vi "运维调试_氨氮.vi"() -> ()   [LabVIEW 2016, in "斯坦道氨氮.lvlib"]
uses:
  <vilib>/Utility/miscctls.llb/LVPointTypeDef.ctl
  <vilib>/Utility/config.llb/NI_LVConfig.lvlib
  <vilib>/ptbypt/NI_PtbyPt.lvlib
panel:
  in  "定时设置":cluster{"启动":bool, "控制命令":T1, "测量参数":T2}(xcontrol)
  in  "仪器参数设置":bool
  in  "模块启用":bool
  in  "串口设置":bool
  in  "备用系数一键写入":bool
  in  "公式一键写入":bool
  in  "流程路径":path=path "C:/Users/STD/Documents/斯坦道流程文件/流程.xml"
  in  "曲线模型":cluster{"X^2":dbl, "X":dbl, "B":dbl, "r^2":dbl}(xcontrol)
  out "字符串":string
  in  "质控参数设置":bool
  in  "自动测试量程配置":T3
  out "温度2":sgl
  out "温度1":sgl
  out "ADC":sgl
  out "固件版本号":string
  in  "数组":string[](array[string])
  in  "备用系数写入":bool
  in  "备用系数读取":bool
  in  "备用系数":T4
  in  "量程切换阈值写入":bool
  in  "量程切换阈值读取":bool
  in  "量程切换阈值":cluster{"阈值":dbl, "标液浓度":dbl}
  in  "参数下拉列表":enum16{"总磷", "总氮", "氨氮"}(ring)=enum."氨氮"
  in  "量程下拉列表":enum16{"低量程", "高量程"}(ring)
  in  "测量模式下拉列表":enum16{"水样测量", "零点核查", "跨度核查", "标样核查", "加标回收"}(ring)
  in  "公式":cluster{"X^2":dbl, "X":dbl, "b":dbl}
  in  "写公式":bool
  in  "读公式":bool
  in  "返回":bool
  in  "设置":bool
  out "序列号":string="序列号"
  out "测量数据":T5(xcontrol)
  out "集成报警信息":string
  out "运行状态":T6(xcontrol)
  in  "停止":bool
  in  "手动启动":bool
  in  "单步测试":bool
  in  "总磷氨氮调试":u16[](xcontrol)
  out "F3":sgl format="%#.6f"
  out "F2":sgl format="%#.6f"
  out "F1":sgl format="%#.6f"
  out "F0":sgl format="%#.6f"
  out "多列列表框":i32(listbox)
  # "参数设置"
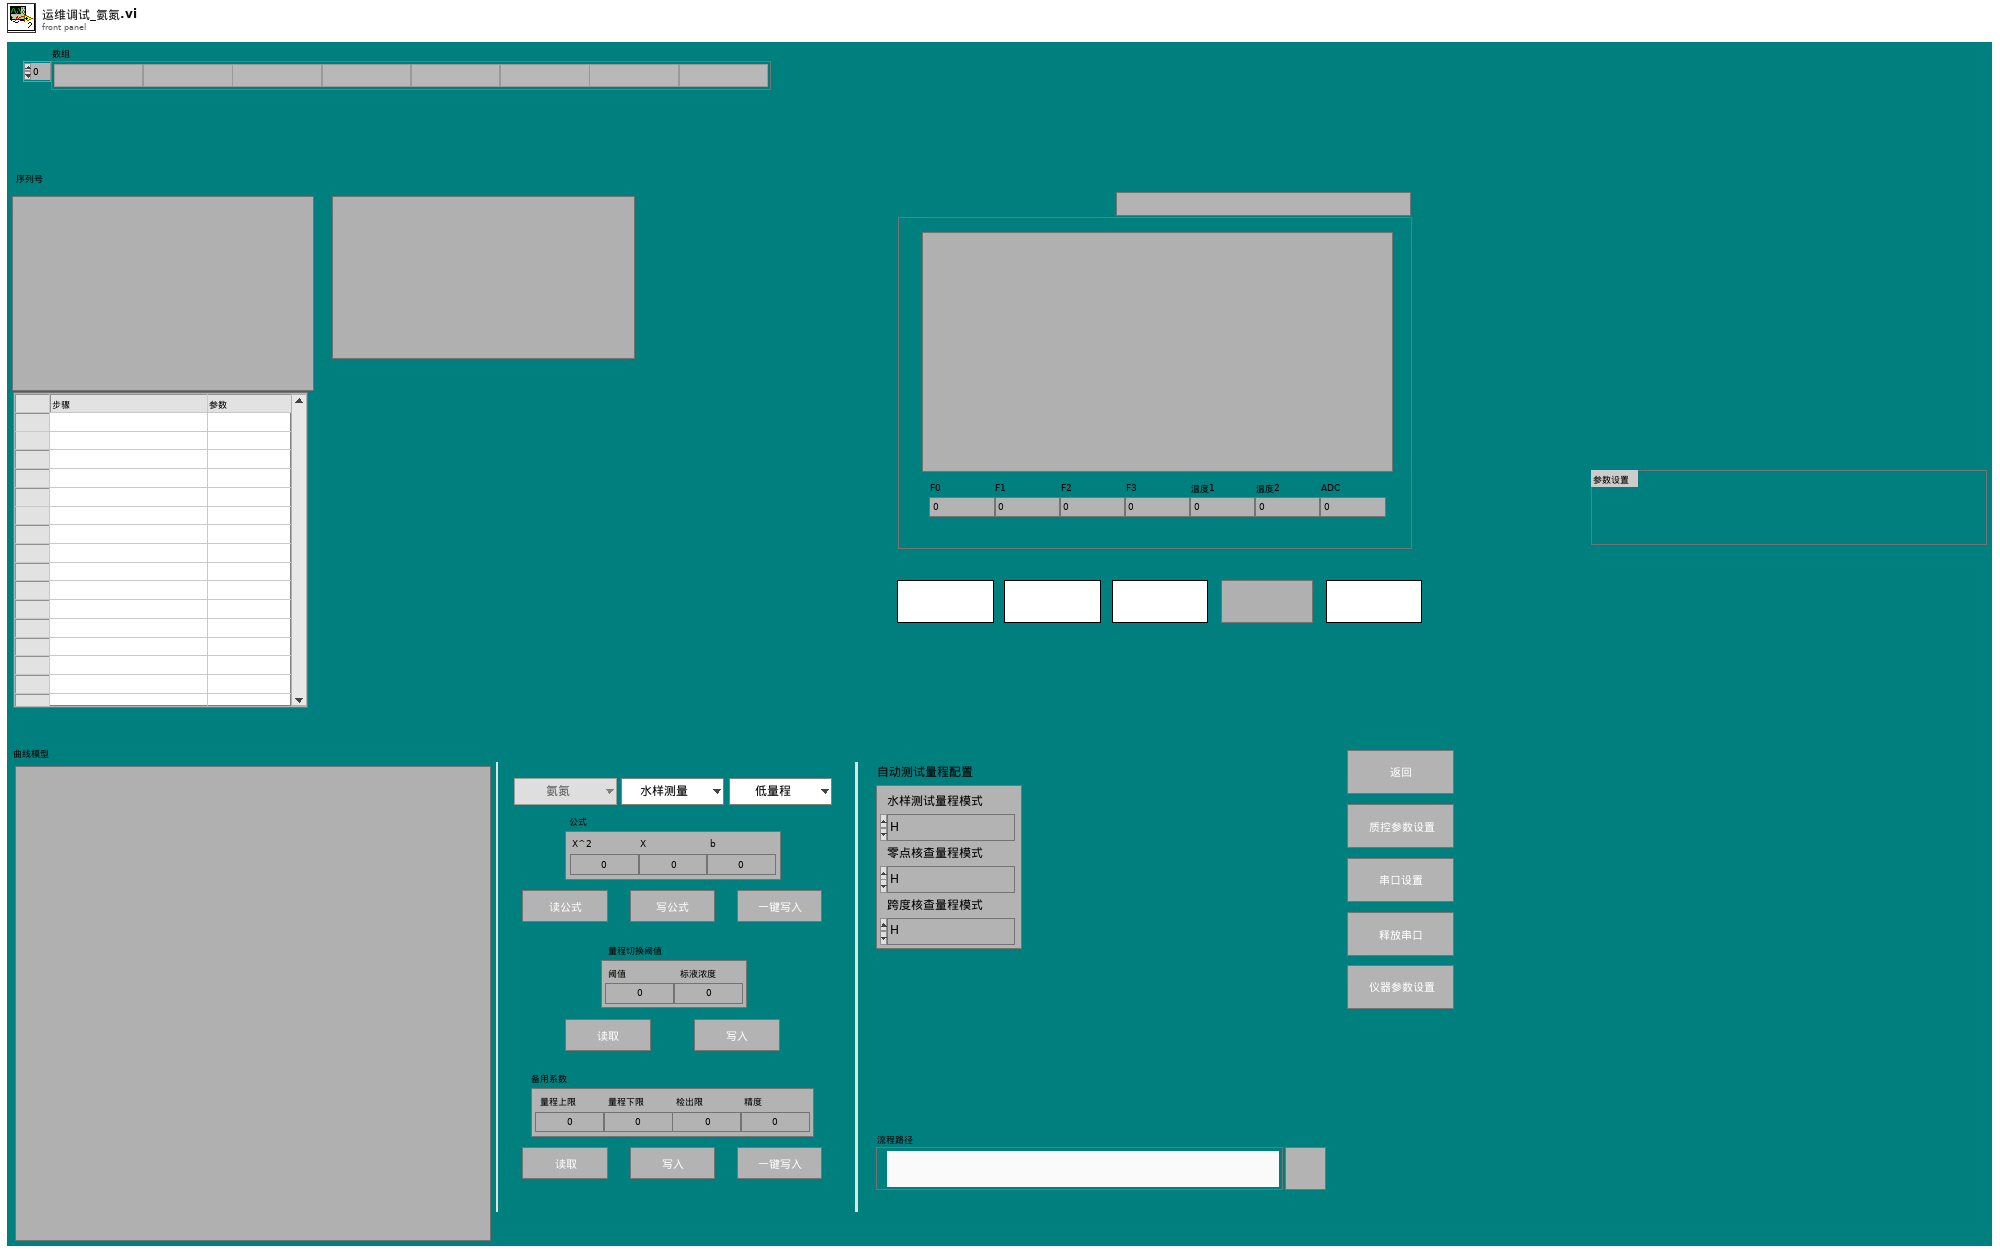
[diagram p1: front panel]
types:
  T1 = typedef "定时设置.xctl/国标控制命令.ctl" = enum16{"启动测量", "标样核查", "零点核查", "跨度核查", "空白测试", "平行样测试", "加标回收", "空白校准", "标样校准", "初始化（清洗）", "停止测试", "仪器重启", "校时", "模式设置", "测量间隔设置"}
  T2 = typedef "定时设置.xctl/测量参数.ctl" = u16
  T3 = cluster{"水样测试量程模式":enum16{"H", "L", "AUTO"}, "空白核查量程模式":enum16{"H", "L", "AUTO"}, "跨度核查量程模式":enum16{"H", "L", "AUTO"}}
  T4 = cluster{"量程上限":dbl, "量程下限":dbl, "检出限":dbl, "精度":dbl}
  T5 = cluster{"flowid":u16, "测量精度":u16, "测量数据区":cluster{"因子编码":u32, "单位":u16, "标样参考值":sgl, "水样数据时间":timestamp, "水样实测值":sgl, "水样数据标识":string, "标样数据时间":timestamp, "标样实测值":sgl, "标样数据标识":string, "空白数据时间":timestamp, "空白实测值":sgl, "空白数据标识":string, "零点核查数据时间":timestamp, "零点核查实测值":sgl, "零点核查数据标识":string, "跨度核查数据时间":timestamp, "跨度核查实测值":sgl, "跨度核查数据标识":string, "加标回收数据时间":timestamp, "加标回收实测值":sgl, "加标回收数据标识":string, "平行样数据时间":timestamp, "平行样实测值":sgl, "平行样数据标识":string, "F0":sgl, "F1":sgl, "F2":sgl, "F3":sgl, "F4":sgl, "F5":sgl, "F6":sgl, "F7":sgl, "温度":sgl, "湿度":sgl, "X值":sgl}}
  T6 = cluster{"系统时间":timestamp, "工作状态":enum16{"空闲", "水样测试", "标样核查", "零点核查", "跨度核查", "空白测试", "平行样测试", "加标回收", "空白校准", "标样校准", "初始化（清洗）"}, "测量模式":enum16{"待机", "连续模式", "周期模式", "定点模式", "受控模式", "手动模式"}, "告警代码":u16, "故障代码":u16, "日志代码":u16, "软件版本":u16, "F0":sgl, "F1":sgl, "F2":sgl, "F3":sgl, "T":sgl, "H":sgl, "id":u16, "flowid":u16, "量程":u16, "总磷控温温度1":sgl, "营养盐控温温度2":sgl, "ADC":sgl}
  T7 = cluster{"时间源选择":enum16{"系统时间源", "仪器时间源"}, "外部时间源":timestamp}
  T8 = enum16{"空闲", "水样测试", "标样核查", "零点核查", "跨度核查", "空白测试", "平行样测试", "加标回收", "空白校准", "标样校准", "初始化（清洗）"}
  T9 = enum32{"Bad", "Idle", "Run top level", "Running"}
  T10 = typedef "LVPointTypeDef.ctl" = cluster{"Horizontal":i16, "Vertical":i16}
  T11 = cluster{"因子编码":u32, "单位":u16, "标样参考值":sgl, "水样数据时间":timestamp, "水样实测值":sgl, "水样数据标识":string, "标样数据时间":timestamp, "标样实测值":sgl, "标样数据标识":string, "空白数据时间":timestamp, "空白实测值":sgl, "空白数据标识":string, "零点核查数据时间":timestamp, "零点核查实测值":sgl, "零点核查数据标识":string, "跨度核查数据时间":timestamp, "跨度核查实测值":sgl, "跨度核查数据标识":string, "加标回收数据时间":timestamp, "加标回收实测值":sgl, "加标回收数据标识":string, "平行样数据时间":timestamp, "平行样实测值":sgl, "平行样数据标识":string, "F0":sgl, "F1":sgl, "F2":sgl, "F3":sgl, "F4":sgl, "F5":sgl, "F6":sgl, "F7":sgl, "温度":sgl, "湿度":sgl, "X值":sgl}
  T12 = typedef "NI_LVConfig.lvlib/Config Data RefNum.ctl" = refnum<k1>
  T13 = cluster{"参数下拉列表":enum16{"总磷", "总氮", "氨氮"}, "测量模式下拉列表":enum16{"水样测量", "零点核查", "跨度核查", "标样核查", "加标回收"}, "量程下拉列表":enum16{"低量程", "高量程"}}
  T14 = cluster{"启动模式":enum16{"跨度核查", "水样测量", "空白核查", "标样核查", "加标回收"}, "启动参数":u16, "量程":enum16{"低量程", "高量程"}}
  T15 = cluster{"时间标识":timestamp, "设备":string, "日志信息":string, "流程参数":string}
  T16 = cluster{"时间标识":timestamp, "设备":string, "日志信息":string}
  T17 = typedef "LVRowAndColumnUnsignedTypeDef.ctl" = cluster{"Row":u32, "Column":u32}
  T18 = cluster{"站号":u16, "量程切换":enum32{"H", "L", "AUTO"}, "控制命令":enum16{"启动测量", "标样核查", "零点核查", "跨度核查", "空白测试", "平行样测试", "加标回收", "空白校准", "标样校准", "初始化（清洗）", "停止测试", "仪器重启", "校时", "模式设置", "测量间隔设置"}, "模式设置":enum16{"待机", "连续模式", "周期模式", "定点模式", "受控模式", "手动模式"}, "测量间隔":u16}
  T19 = cluster{"氨氮跨度值":dbl, "氨氮零点标准液浓度":dbl, "氨氮跨度标准液浓度":dbl, "氨氮标准液标准浓度":dbl}
  T20 = cluster{"确定":bool, "跨度值":dbl, "零点标准液浓度":dbl, "跨度标准液浓度":dbl, "标准液标准浓度":dbl}
  T21 = cluster{"测量量程":dbl, "测量精度":dbl, "测量间隔":dbl, "消解温度":dbl, "消解时长":dbl, "空白校准时间":timestamp, "曲线截距":dbl, "曲线斜率":dbl, "测量检出限":dbl, "测量信号值":dbl, "线性相关系数":dbl, "二次多项式系数":dbl, "标样校准时间":timestamp, "稀释倍数":dbl, "三项式系数":dbl, "空白标定系数":dbl, "量程系数":dbl, "F0/ORPA":dbl, "F1/ORPB":dbl, "F2/ORPK":dbl, "F3":dbl, "F4":dbl, "F5":dbl, "F6":dbl, "F7":dbl, "X0/滴定数":dbl, "量程":dbl}
  T22 = cluster{"确定":bool, "测量量程":dbl, "测量精度":dbl, "测量间隔":dbl, "消解温度":dbl, "消解时长":dbl, "空白校准时间":timestamp, "曲线截距":dbl, "曲线斜率":dbl, "测量检出限":dbl, "测量信号值":dbl, "线性相关系数":dbl, "二次多项式系数":dbl, "标样校准时间":timestamp, "稀释倍数":dbl, "三项式系数":dbl, "空白标定系数":dbl, "量程系数":dbl, "F0/ORPA":dbl, "F1/ORPB":dbl, "F2/ORPK":dbl, "F3":dbl, "F4":dbl, "F5":dbl, "F6":dbl, "F7":dbl, "X0/滴定数":dbl, "量程":dbl}
  T23 = enum8{"Enabled", "Disabled", "Disabled and Grayed Out"}
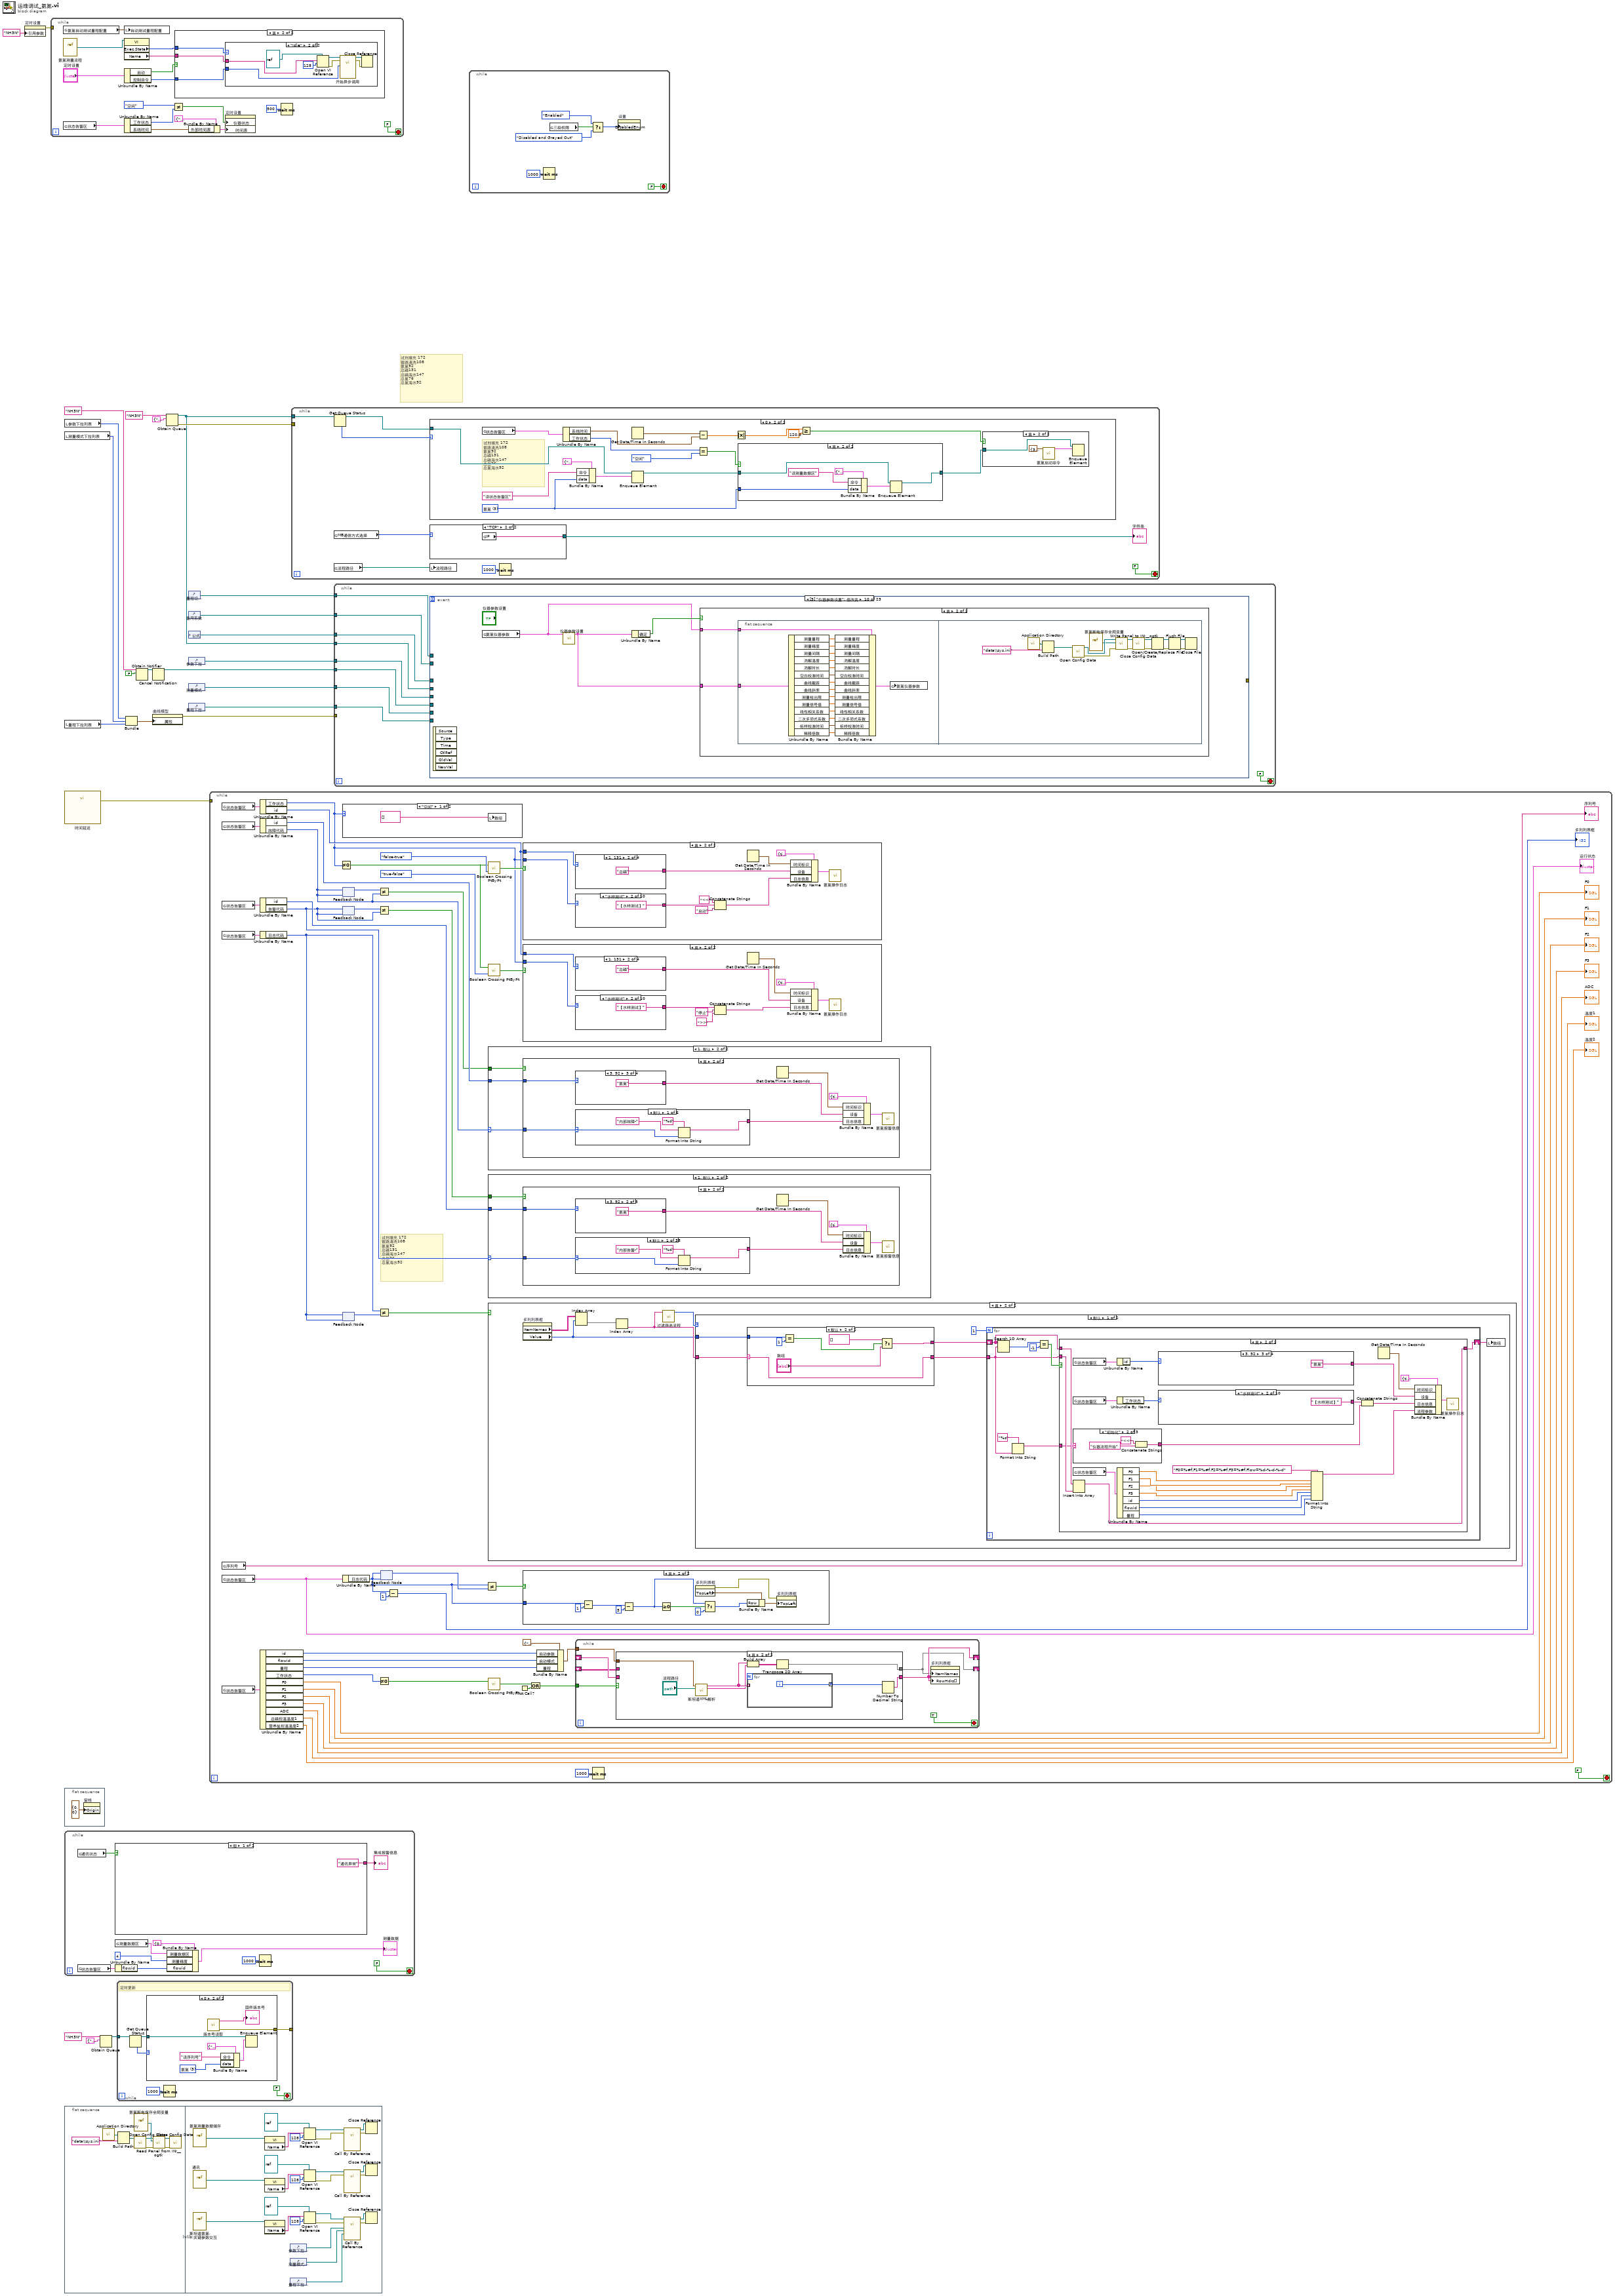
[diagram p0: block diagram]
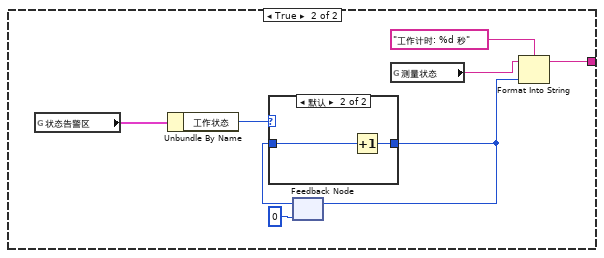
[diagram p3: hidden frame]
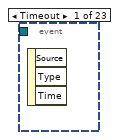
[diagram p7: hidden frame]
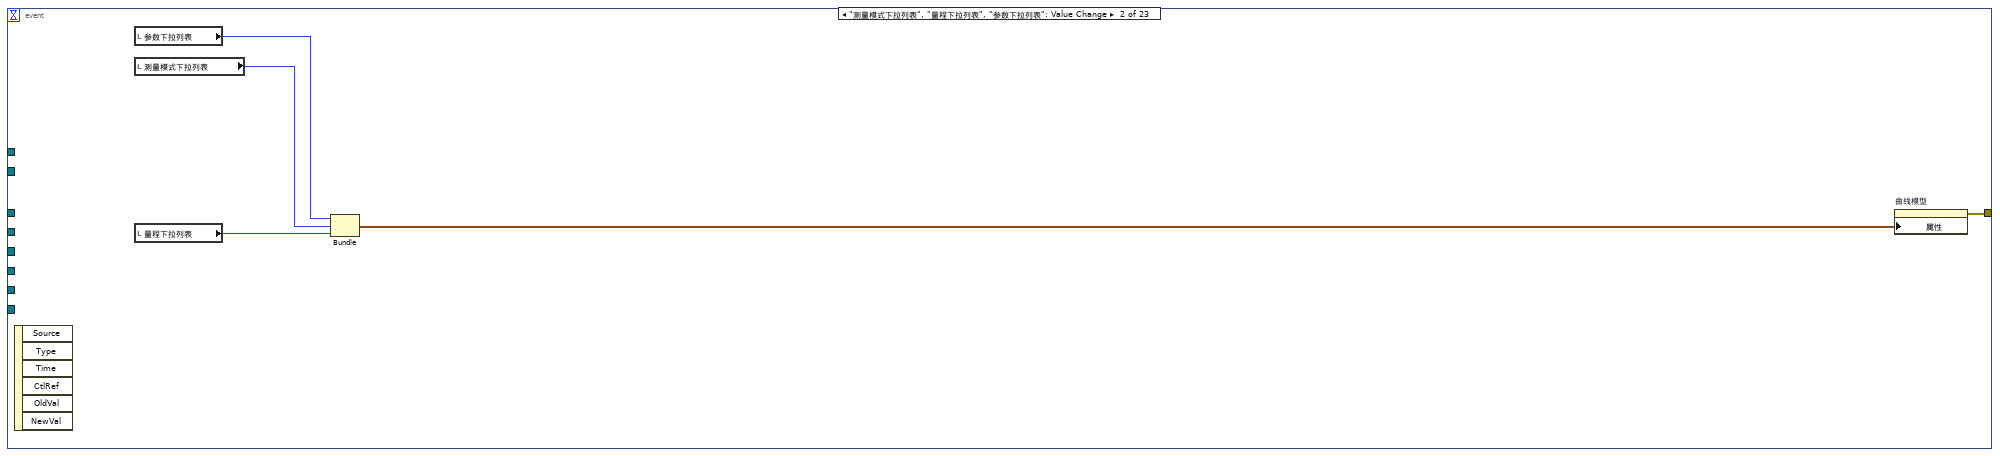
[diagram p8: hidden frame]
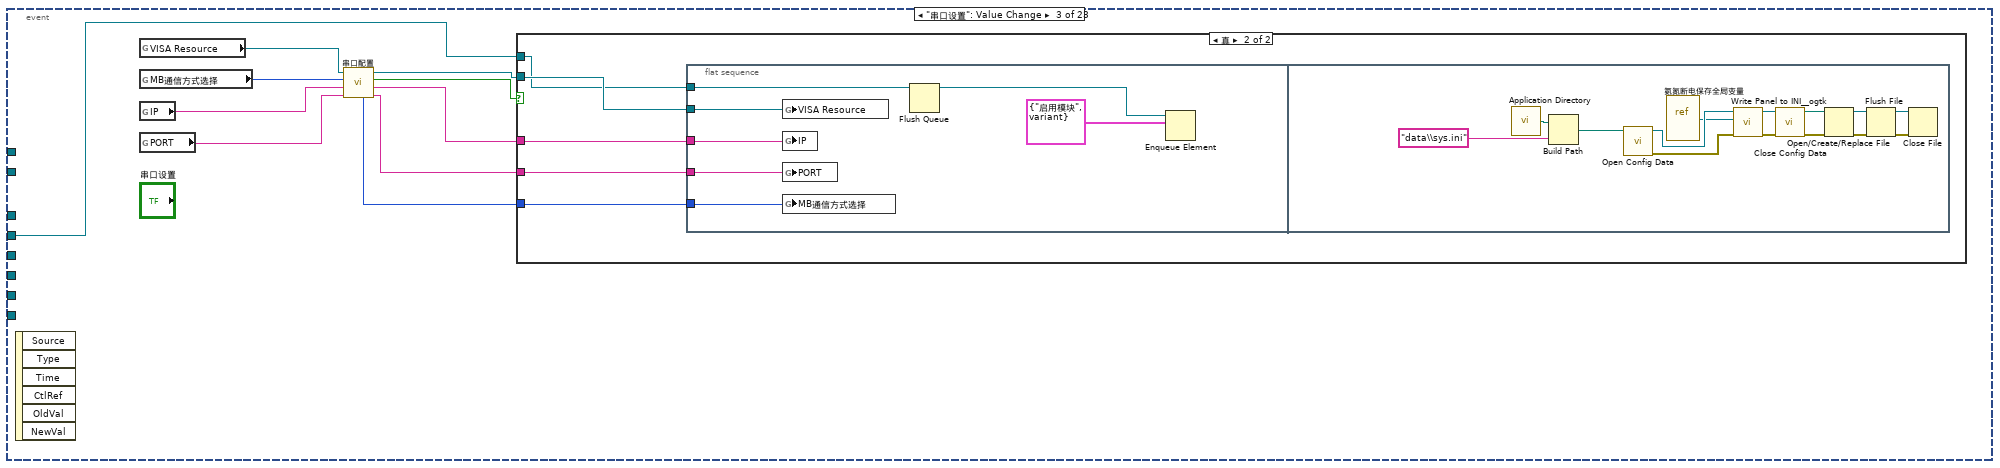
[diagram p9: hidden frame]
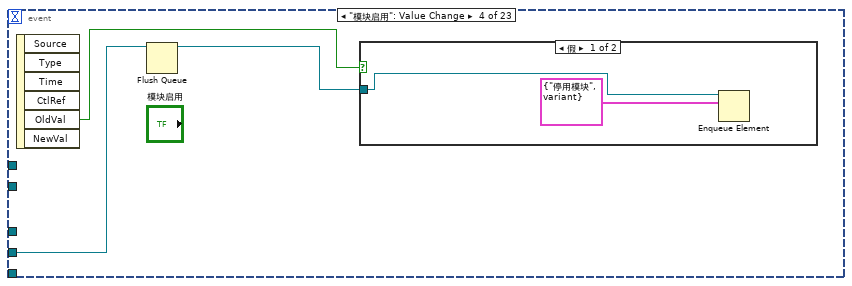
[diagram p11: hidden frame]
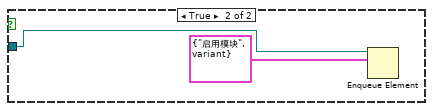
[diagram p12: hidden frame]
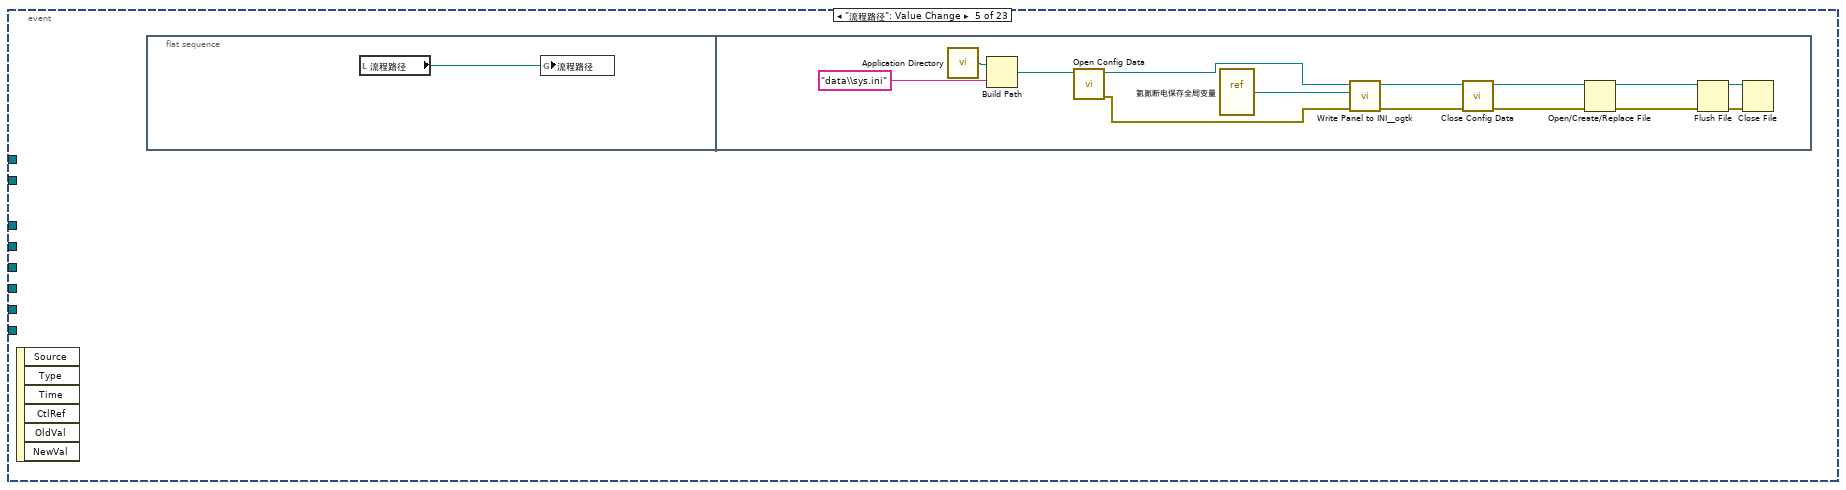
[diagram p13: hidden frame]
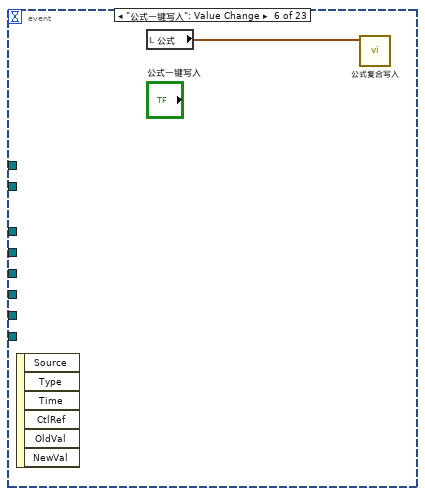
[diagram p14: hidden frame]
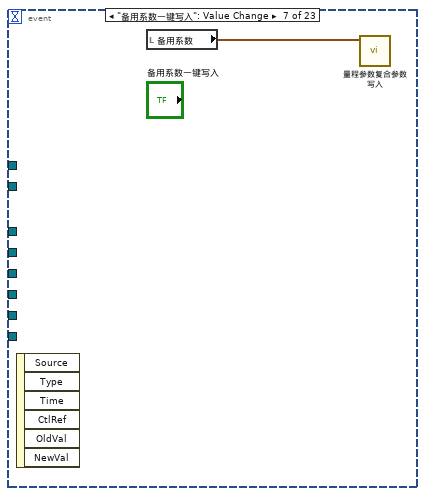
[diagram p15: hidden frame]
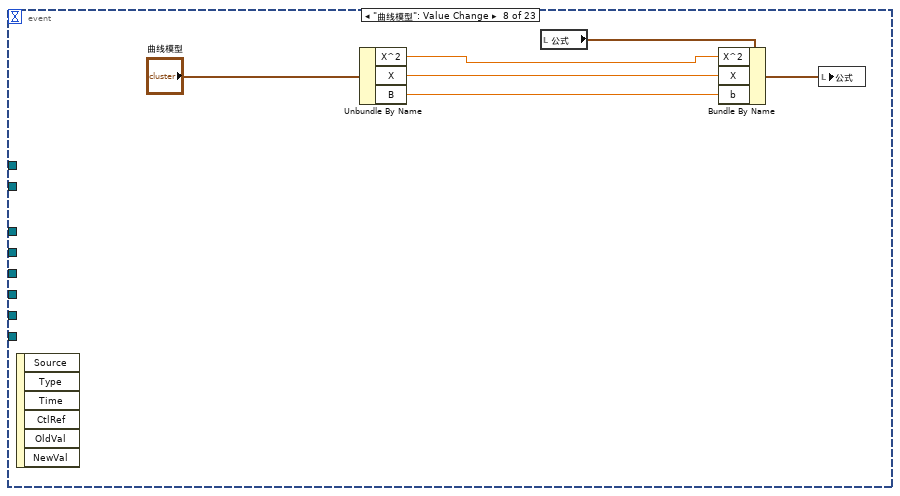
[diagram p16: hidden frame]
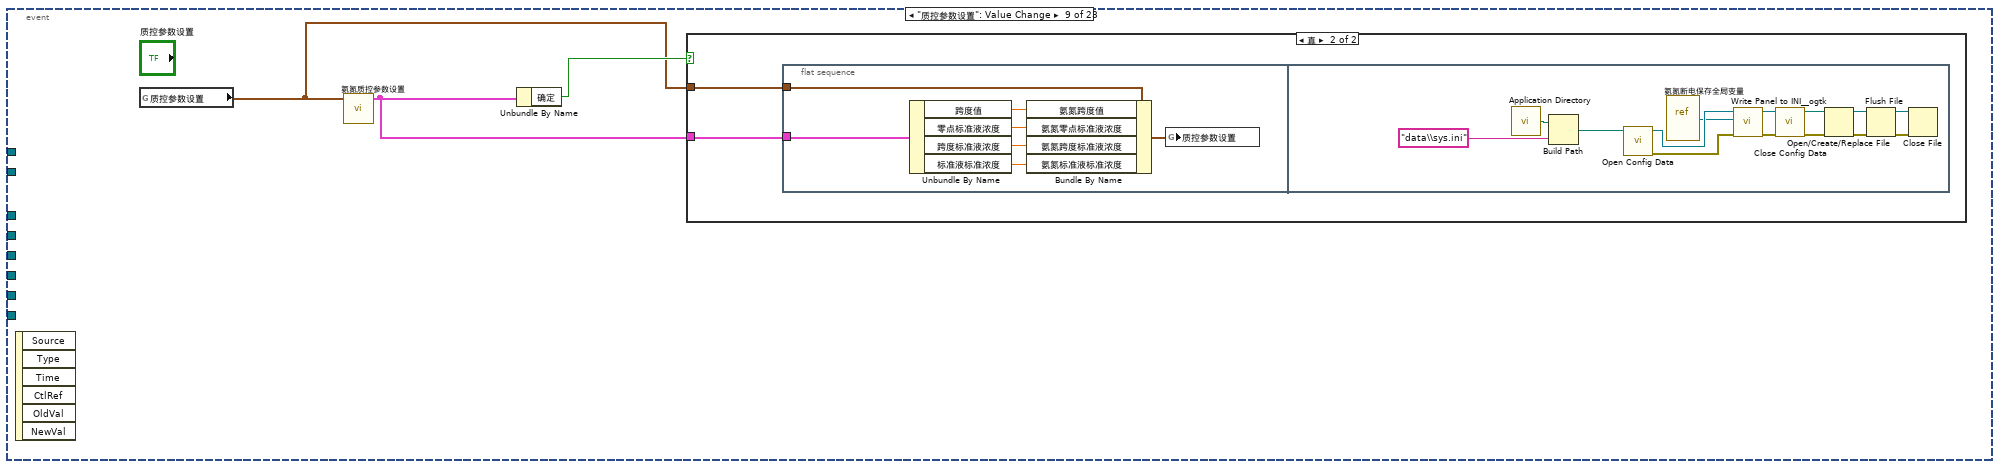
[diagram p17: hidden frame]
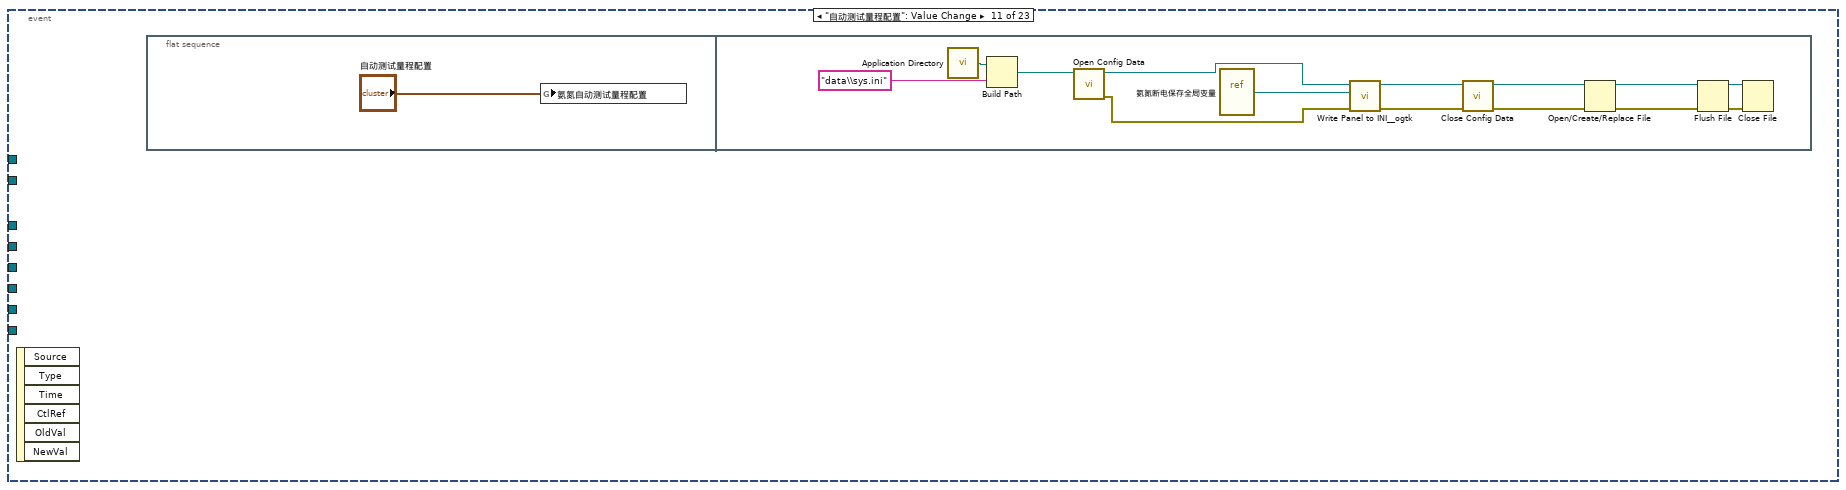
[diagram p20: hidden frame]
diagram:
  # "试剂填充 172 \n管路清洗108\n氨氮92\n总磷131\n总磷海水147\n总氮76\n总氮海水92"
  n1 = property on="定时设置" class="定时设置 (严格)"("引用参数"="NH3N") -> (error out=w1:errorcluster)  [unwired: 2 in, 1 out]
  n2 = while {
    tunnel: w1 -> [_]
    stop <- FALSE stop-if-true
    n3 = global read "氨氮断电保存全局变量.vi" "氨氮自动测试量程配置"() -> (w39:T3)
    n4 = vi-ref "氨氮测量流程.vi"() -> (w38:refnum<vi>)
    n5 = global read "VAR氨氮全局变量.vi" "状态告警区"() -> (w32:T6)
    n6 = local write "自动测试量程配置"(w39) -> ()
    n7 = property class="VI"(reference=w38) -> ("Exec.State"=w37:T9, "Name"=w36:string)  [unwired: 1 in, 2 out]
    n8 = Unbundle By Name("定时设置") -> ("启动"=w34:bool, "控制命令"=w33:T1)
    n9 = Unbundle By Name(w32) -> ("工作状态"=w31:T8, "系统时间"=w26:timestamp)
    n10 = Not Equal?(x=T8."空闲", y=w31) -> (x != y?=w29:bool)
    n11 = case shown="真" w34 {
      tunnel: w36 -> [_ w44]
      tunnel: w37 -> [_ w43]
      tunnel: w33 -> [_ w42]
      frame False {
      }
      frame True {
        n12 = case shown="\"Idle\"" w43 {
          tunnel: w44 -> [_ w48]
          tunnel: w42 -> [_ w45]
          frame "Bad", Default {
          }
          frame "Idle" {
            n13 = Open VI Reference(type specifier VI Refnum (for type only)=refnum<vi> refnum, vi path=w48, options=128 ("选项")) -> (vi reference=w49:refnum<vi>, error out=w50:errorcluster)  [unwired: 3 in]
            n14 = call-by-ref "开始异步调用"(reference=w49, error in=w50, "控制命令"=w45) -> (reference out=w51:refnum<vi>, error out=w52:errorcluster)  [unwired: 11 in]
            n15 = Close Reference(reference=w51, error in (no error)=w52) -> ()  [unwired: 1 out]
          }
        }
      }
    }
    n16 = Bundle By Name(cluster=T7 {"时间源选择"=enum."仪器时间源", "外部时间源"=timestamp(0 s since 1904-01-01)} ("时间源"), "外部时间源"=w26) -> (w27:T7)
    n17 = property on="定时设置" class="定时设置 (严格)"("仪器状态"=w29, "时间源"=w27) -> ()  [unwired: 2 in, 2 out]
    n18 = Wait (ms)(milliseconds to wait=u32 500 ("等待时间（毫秒）")) -> ()  [unwired: 1 out]
  }
  n19 = local read "参数下拉列表"() -> (w6:enum16{"总磷", "总氮", "氨氮"})
  n20 = local read "测量模式下拉列表"() -> (w5:enum16{"水样测量", "零点核查", "跨度核查", "标样核查", "加标回收"})
  n21 = local read "量程下拉列表"() -> (w4:enum16{"低量程", "高量程"})
  n22 = call "时间延迟"() -> ("error out"=w15:errorcluster)  [unwired: 11 in]
  n23 = flat-sequence {
    frame #0 {
      n24 = property on="窗格" class="Pane"("Origin"=T10 {"Horizontal"=0, "Vertical"=0} ("原点")) -> ()  [unwired: 2 in, 2 out]
    }
  }
  n25 = while {
    stop <- FALSE stop-if-true
    n26 = global read "VAR氨氮全局变量.vi" "通讯状态"() -> (w61:bool)
    n27 = global read "VAR氨氮全局变量.vi" "状态告警区"() -> (w59:T6)
    n28 = case shown="假" w61 {
      tunnel: ["通讯异常" ("集成报警信息") w66] -> w60
      frame False {
      }
      frame True {
        n29 = global read "VAR氨氮全局变量.vi" "状态告警区"() -> (w72:T6)
        n30 = Unbundle By Name(w72) -> ("工作状态"=w71:T8)
        n31 = feedback #1(0) -> (w69:i32)
        n32 = case shown="默认" w71 {
          tunnel: w69 -> [_ w74]
          tunnel: [_ w73] -> w67
          frame "空闲" {
          }
          frame Default {
            n33 = Increment(x=w74) -> (x+1=w73:i32)
          }
        }
        n34 = feedback-in #1(w67) -> ()
        n35 = global read "VAR氨氮全局变量.vi" "测量状态"() -> (w65:string)
        n36 = Format Into String(format string="工作计时: %d 秒" ("格式字符串"), initial string=w65, w67) -> (resulting string=w66:string)  [unwired: 1 in, 1 out]
      }
    }
    "集成报警信息" <- w60
    n37 = global read "VAR氨氮全局变量.vi" "测量数据区"() -> (w54:T11)
    n38 = Unbundle By Name(w59) -> ("flowid"=w58:u16)
    n39 = Bundle By Name(cluster=T5 {"flowid"=0, "测量精度"=0, "测量数据区"={"因子编码"=0, "单位"=0, "标样参考值"=0.0, "水样数据时间"=timestamp(0 s since 1904-01-01), "水样实测值"=0.0, "水样数据标识"="", "标样数据时间"=timestamp(0 s since 1904-01-01), "标样实测值"=0.0, "标样数据标识"="", "空白数据时间"=timestamp(0 s since 1904-01-01), "空白实测值"=0.0, "空白数据标识"="", "零点核查数据时间"=timestamp(0 s since 1904-01-01), "零点核查实测值"=0.0, "零点核查数据标识"="", "跨度核查数据时间"=timestamp(0 s since 1904-01-01), "跨度核查实测值"=0.0, "跨度核查数据标识"="", "加标回收数据时间"=timestamp(0 s since 1904-01-01), "加标回收实测值"=0.0, "加标回收数据标识"="", "平行样数据时间"=timestamp(0 s since 1904-01-01), "平行样实测值"=0.0, "平行样数据标识"="", "F0"=0.0, "F1"=0.0, "F2"=0.0, "F3"=0.0, "F4"=0.0, "F5"=0.0, "F6"=0.0, "F7"=0.0, "温度"=0.0, "湿度"=0.0, "X值"=0.0}} ("总氮测量数据"), "测量数据区"=w54, "测量精度"=u16 4, "flowid"=w58) -> (→"测量数据":T5)
    n40 = Wait (ms)(milliseconds to wait=u32 1000 ("等待时间（毫秒）")) -> ()  [unwired: 1 out]
  }
  n41 = flat-sequence {
    frame #0 {
      n42 = call <vilib>:"Application Directory.vi"() -> ("Application Directory"=w82:path)
      n43 = Build Path(base path=w82, name or relative path="data\\sys.ini" ("名称或相对路径")) -> (appended path=w80:path)
      n44 = vi-ref "氨氮断电保存全局变量.vi"() -> (w78:refnum<vi>)
      n45 = call <vilib>:"Open Config Data.vi"("configuration file path"=w80) -> ("error out"=w76:errorcluster, "refnum"=w79:T12)  [unwired: 8 in, 1 out]
      n46 = call <userlib>:"Read Panel from INI__ogtk.vi"("error in (no error)"=w76, "VI ref"=w78, "refnum"=w79) -> ("error out"=w75:errorcluster, "refnum out"=w77:T12)  [unwired: 7 in]
      n47 = call <vilib>:"Close Config Data.vi"("error in (no error)"=w75, "refnum"=w77) -> ()  [unwired: 8 in, 2 out]
    }
    frame #1 {
      n48 = vi-ref "氨氮测量数据储存.vi"() -> (w101:refnum<vi>)
      n49 = vi-ref "通讯.vi"() -> (w109:refnum<vi>)
      n50 = vi-ref "斯坦道氨氮.lvlib:关键参数交互.vi"() -> (w86:refnum<vi>)
      n51 = property class="VI"(reference=w101) -> ("Name"=w94:string)  [unwired: 1 in, 2 out]
      n52 = property class="VI"(reference=w109) -> ("Name"=w108:string)  [unwired: 1 in, 2 out]
      n53 = property class="VI"(reference=w86) -> ("Name"=w93:string)  [unwired: 1 in, 2 out]
      n54 = control-ref of="参数下拉列表"() -> (w85:refnum<vi>)
      n55 = control-ref of="测量模式下拉列表"() -> (w84:refnum<vi>)
      n56 = control-ref of="量程下拉列表"() -> (w83:refnum<vi>)
      n57 = Open VI Reference(type specifier VI Refnum (for type only)=refnum<vi> refnum, vi path=w94, options=128 ("选项")) -> (vi reference=w96:refnum<vi>, error out=w98:errorcluster)  [unwired: 3 in]
      n58 = Open VI Reference(type specifier VI Refnum (for type only)=refnum<vi> refnum, vi path=w108, options=128 ("选项")) -> (vi reference=w106:refnum<vi>, error out=w104:errorcluster)  [unwired: 3 in]
      n59 = Open VI Reference(type specifier VI Refnum (for type only)=refnum<vi> refnum, vi path=w93, options=128 ("选项")) -> (vi reference=w91:refnum<vi>, error out=w89:errorcluster)  [unwired: 3 in]
      n60 = call-by-ref "?"(reference=w96, error in=w98) -> (reference out=w100:refnum<vi>, error out=w99:errorcluster)  [unwired: 12 in]
      n61 = call-by-ref "?"(reference=w106, error in=w104) -> (reference out=w102:refnum<vi>, error out=w103:errorcluster)  [unwired: 12 in]
      n62 = call-by-ref "?"(reference=w91, error in=w89, "量程下拉列表"=w83, "测量模式下拉列表"=w84, "参数下拉列表"=w85) -> (reference out=w87:refnum<vi>, error out=w88:errorcluster)  [unwired: 9 in]
      n63 = Close Reference(reference=w100, error in (no error)=w99) -> ()  [unwired: 1 out]
      n64 = Close Reference(reference=w102, error in (no error)=w103) -> ()  [unwired: 1 out]
      n65 = Close Reference(reference=w87, error in (no error)=w88) -> ()  [unwired: 1 out]
    }
  }
  n66 = Obtain Queue(name (unnamed)="NH3N" ("名称（未命名）"), element data type=cluster{"命令":string, "data":variant} {"命令"="", "data"=variant}) -> (queue out=w12:refnum<queue>)  [unwired: 3 in, 2 out]
  n67 = while {
    tunnel: w12 -> [w114]
    tunnel: [w112] -> _
    stop <- FALSE stop-if-true
    # "定时更新"
    n68 = Get Queue Status(queue=w114) -> (queue out=w111:refnum<queue>, # elements in queue=w110:i32)  [unwired: 2 in, 6 out]
    n69 = case shown="0" w110 {
      tunnel: [_ w117] -> w112
      tunnel: w111 -> [_ w116]
      frame Default {
      }
      frame 0 {
        w120 = u16 3 items=["总磷"=1, "氨氮"=3] ("站号")
        n70 = call "版本号读取.vi"() -> ("error out"=w117:errorcluster, "固件版本号"=→"固件版本号":string)  [unwired: 10 in]
        n71 = Bundle By Name(cluster=cluster{"命令":string, "data":variant} {"命令"="", "data"=variant} ("元素"), "命令"="读序列号", "data"=w120) -> (w119:cluster{"命令":string, "data":variant})
        n72 = Enqueue Element(queue=w116, element=w119) -> ()  [unwired: 2 in, 3 out]
      }
    }
    n73 = Wait (ms)(milliseconds to wait=u32 1000 ("等待时间（毫秒）")) -> ()  [unwired: 1 out]
  }
  n74 = Bundle("参数下拉列表"=w6, "测量模式下拉列表"=w5, "量程下拉列表"=w4) -> (w3:T13)  [unwired: 1 in]
  n75 = Obtain Notifier(name (unnamed)="NH3N" ("名称（未命名）"), notification data type=FALSE) -> (notifier out=w8:refnum<notifier>)  [unwired: 2 in, 2 out]
  n76 = Cancel Notification(0:w8) -> (8:w7:refnum<notifier>)  [unwired: 1 in, 2 out]
  n77 = property on="曲线模型" class="曲线模型 (严格)"("属性"=w3) -> (error out=w11:errorcluster)  [unwired: 2 in, 1 out]
  n78 = Obtain Queue(name (unnamed)="NH3N" ("名称（未命名）"), element data type=cluster{"命令":string, "data":variant} {"命令"="", "data"=variant}) -> (queue out=w22:refnum<queue>, error out=w23:errorcluster)  [unwired: 3 in, 1 out]
  n79 = control-ref of="量程切换阈值"() -> (w17:refnum<vi>)
  n80 = control-ref of="备用系数"() -> (w16:refnum<vi>)
  n81 = control-ref of="公式"() -> (w18:refnum<vi>)
  n82 = control-ref of="参数下拉列表"() -> (w20:refnum<vi>)
  n83 = control-ref of="测量模式下拉列表"() -> (w19:refnum<vi>)
  n84 = control-ref of="量程下拉列表"() -> (w21:refnum<vi>)
  n85 = while {
    tunnel: w15 -> [_]
    stop <- FALSE stop-if-true
    # "试剂填充 172 \n管路清洗108\n氨氮92\n总磷131\n总磷海水147\n总氮76\n总氮海水92"
    n86 = global read "VAR氨氮全局变量.vi" "状态告警区"() -> (w143:T6)
    n87 = global read "VAR氨氮全局变量.vi" "状态告警区"() -> (w148:T6)
    n88 = global read "VAR氨氮全局变量.vi" "状态告警区"() -> (w153:T6)
    n89 = global read "VAR氨氮全局变量.vi" "状态告警区"() -> (w141:T6)
    n90 = global read "VAR氨氮全局变量.vi" "序列号"() -> (→"序列号":string)
    n91 = global read "VAR氨氮全局变量.vi" "状态告警区"() -> (w156:T6)
    "运行状态" <- w156
    n92 = global read "VAR氨氮全局变量.vi" "状态告警区"() -> (w164:T6)
    n93 = Unbundle By Name(w143) -> ("工作状态"=w123:T8, "id"=w124:u16)
    n94 = Unbundle By Name(w148) -> ("id"=w147:u16, "故障代码"=w144:u16)
    n95 = Unbundle By Name(w153) -> ("id"=w152:u16, "告警代码"=w149:u16)
    n96 = Unbundle By Name(w141) -> ("日志代码"=w140:u16)
    n97 = Unbundle By Name(w164) -> ("id"=w161:u16, "flowid"=w163:u16, "量程"=w162:u16, "工作状态"=w131:T8, "F0"=→"F0":sgl, "F1"=→"F1":sgl, "F2"=→"F2":sgl, "F3"=→"F3":sgl, "ADC"=→"ADC":sgl, "总磷控温温度1"=→"温度1":sgl, "营养盐控温温度2"=→"温度2":sgl)
    n98 = Not Equal To 0?(x=w123) -> (x != 0?=w126:bool)
    n99 = case shown="\"空闲\"" w123 {
      frame "空闲" {
        n100 = local write "数组"(string[] [] ("数组")) -> ()
      }
      frame "水样测试", Default {
      }
    }
    n101 = feedback #2(w144) -> (w145:u16)
    n102 = feedback-in #2(w144) -> ()
    n103 = feedback #3(w149) -> (w150:u16)
    n104 = feedback-in #3(w149) -> ()
    n105 = feedback #4(w140) -> (w142:u16)
    n106 = feedback-in #4(w140) -> ()
    n107 = Unbundle By Name(w156) -> ("日志代码"=w137:u16)
    n108 = Not Equal?(x=w145, y=w144) -> (x != y?=w146:bool)
    n109 = Not Equal?(x=w150, y=w149) -> (x != y?=w151:bool)
    n110 = Not Equal?(x=w140, y=w142) -> (x != y?=w139:bool)
    n111 = Not Equal To 0?(x=w131) -> (x != 0?=w166:bool)
    n112 = feedback-in #5(w137) -> ()
    n113 = feedback #5(w137) -> (w169:u16)
    n114 = Subtract(x=w137, y=1) -> (x-y=→"多列列表框":i32)
    n115 = Not Equal?(x=w137, y=w169) -> (x != y?=w168:bool)
    n116 = call <vilib>:"Boolean Crossing PtByPt.vi"("direction"=enum16{"either", "false-true", "true-false"}."false-true", "input"=w126) -> ("crossing"=w128:bool)  [unwired: 1 in]
    n117 = call <vilib>:"Boolean Crossing PtByPt.vi"("direction"=enum16{"either", "false-true", "true-false"}."true-false", "input"=w126) -> ("crossing"=w125:bool)  [unwired: 1 in]
    n118 = case shown="1, 默认" w144 {
      selector: w144 -> [_ w291]
      tunnel: w147 -> [_ w292]
      tunnel: w146 -> [_ w290]
      frame 0 {
      }
      frame 1, Default {
        n119 = case shown="真" w290 {
          tunnel: w292 -> [_ w299]
          tunnel: w291 -> [_ w294]
          frame False {
          }
          frame True {
            n120 = case shown="3, 92" w299 {
              tunnel: [_ "总磷" ("table输入") "氨氮" ("table输入") "总氮" ("table输入")] -> w295
              frame Default {
              }
              frame 1, 131 {
              }
              frame 3, 92 {
              }
              frame 2, 76 {
              }
            }
            n121 = case shown="默认" w294 {
              selector: w294 -> [w301 _ _ _ _ _]
              tunnel: [w300 "无故障" "电机故障" "温度故障" "通讯故障" "滴定故障"] -> w293
              frame Default {
                n122 = Format Into String(format string="%d" ("格式字符串"), initial string="内部故障-" ("工作状态"), w301) -> (resulting string=w300:string)  [unwired: 1 in, 1 out]
              }
              frame 0 {
              }
              frame 1 {
              }
              frame 2 {
              }
              frame 3 {
              }
              frame 4 {
              }
            }
            n123 = Get Date/Time In Seconds() -> (seconds since 1Jan1904=w296:timestamp)
            n124 = Bundle By Name(cluster=T16 {"时间标识"=timestamp(0 s since 1904-01-01), "设备"="", "日志信息"=""} ("data in"), "时间标识"=w296, "设备"=w295, "日志信息"=w293) -> (w297:T16)
            n125 = call "氨氮报警信息.vi"("data in"=w297) -> ()  [unwired: 10 in, 1 out]
          }
        }
      }
    }
    n126 = case shown="1, 默认" w149 {
      selector: w149 -> [_ w313]
      tunnel: w152 -> [_ w314]
      tunnel: w151 -> [_ w312]
      frame 0 {
      }
      frame 1, Default {
        n127 = case shown="真" w312 {
          tunnel: w314 -> [_ w321]
          tunnel: w313 -> [_ w315]
          frame False {
          }
          frame True {
            n128 = case shown="3, 92" w321 {
              tunnel: ["总磷" ("table输入") "氨氮" ("table输入") "总氮" ("table输入")] -> w317
              frame 1, 131 {
              }
              frame 3, 92 {
              }
              frame 2, 76, Default {
              }
            }
            n129 = case shown="默认" w315 {
              selector: w315 -> [w323 _ _ _ _ _ _ _ _ _ _ _ _ _ _ _ _ _ _ _ _ _ _ _ _ _ _ _ _ _ _ _ _ _ _ _ _ _]
              tunnel: [w322 "无告警" "缺试剂告警" "缺水样告警" "缺蒸馏水告警" "缺标液告警" "仪表漏液告警" "标定异常告警" "超量程告警" "加热异常" "低试剂预警" "超上限告警" "超下限告警" "仪表内部其他异常" "滴定异常告警" "电极异常告警" "量程切换告警" "参数设置告警" "PH电极电位异常" "电导率电极异常" "浊度光度异常" "溶解氧电极异常" "溶解氧光强异常" "温度异常告警" "PH异常告警" "溶解氧异常告警" "电导率异常告警" "浊度异常告警" "叶绿素异常告警" "藻密度异常告警" "蓝绿藻异常告警" "ORP异常告警" "氨氮异常告警" "清洁刷异常告警" "SD卡异常告警" "蓝牙异常告警" "WiFi异常告警" "流程异常告警"] -> w316
              frame Default {
                n130 = Format Into String(format string="%d" ("格式字符串"), initial string="内部告警-" ("工作状态"), w323) -> (resulting string=w322:string)  [unwired: 1 in, 1 out]
              }
              frame 0 {
              }
              frame 1 {
              }
              frame 2 {
              }
              frame 3 {
              }
              frame 4 {
              }
              frame 5 {
              }
              frame 6 {
              }
              frame 7 {
              }
              frame 8 {
              }
              frame 9 {
              }
              frame 10 {
              }
              frame 11 {
              }
              frame 12 {
              }
              frame 13 {
              }
              frame 14 {
              }
              frame 15 {
              }
              frame 16 {
              }
              frame 17 {
              }
              frame 18 {
              }
              frame 19 {
              }
              frame 20 {
              }
              frame 21 {
              }
              frame 22 {
              }
              frame 23 {
              }
              frame 24 {
              }
              frame 25 {
              }
              frame 26 {
              }
              frame 27 {
              }
              frame 28 {
              }
              frame 29 {
              }
              frame 30 {
              }
              frame 31 {
              }
              frame 32 {
              }
              frame 33 {
              }
              frame 34 {
              }
              frame 35 {
              }
              frame 36 {
              }
            }
            n131 = Get Date/Time In Seconds() -> (seconds since 1Jan1904=w318:timestamp)
            n132 = Bundle By Name(cluster=T16 {"时间标识"=timestamp(0 s since 1904-01-01), "设备"="", "日志信息"=""} ("data in"), "时间标识"=w318, "设备"=w317, "日志信息"=w316) -> (w319:T16)
            n133 = call "氨氮报警信息.vi"("data in"=w319) -> ()  [unwired: 10 in, 1 out]
          }
        }
      }
    }
    n134 = case shown="真" w139 {
      frame False {
      }
      frame True {
        n135 = property on="多列列表框" class="MCListbox (严格)"() -> ("ItemNames"=w221:string[][], "Value"=w217:i32)  [unwired: 2 in, 2 out]
        n136 = Index Array(array=w221, index (row)=w217) -> (element=w220:string[])  [unwired: 1 in]
        n137 = Index Array(array=w220) -> (element=w219:string)  [unwired: 1 in]
        n138 = call "过滤筛选流程.vi"("字符串"=w219) -> ("匹配后偏移量"=w218:i32)  [unwired: 10 in]
        n139 = case shown="默认" w218 {
          tunnel: w219 -> [w223 _]
          tunnel: w217 -> [w222 _]
          frame Default {
            n140 = case shown="默认" w223 {
              selector: w223 -> [w229 w236]
              tunnel: [w229 w236] -> w225
              tunnel: [string[] [] ("数组") w231] -> w224
              tunnel: w222 -> [_ w235]
              frame "读数" {
              }
              frame Default {
                n141 = Equal?(x=w235, y=1) -> (x = y?=w233:bool)
                n142 = Select(t=string[] [], s=w233, f="数组") -> (s? t:f=w231:string[])
              }
            }
            n143 = for {
              N: 1 -> [_]
              tunnel: w225 -> [w238]
              shift-right: [w237] -> w226
              shift-left: w224 -> [w239]
              n144 = Search 1D Array(1D array=w239, element=w238) -> (index of element=w242:i32)  [unwired: 1 in]
              n145 = Format Into String(format string="%s" ("格式字符串"), w238) -> (resulting string=w243:string)  [unwired: 2 in, 1 out]
              n146 = Equal?(x=w242, y=-1) -> (x = y?=w240:bool)
              n147 = case shown="真" w240 {
                tunnel: w243 -> [_ w251]
                tunnel: w239 -> [w245 w255]
                tunnel: w238 -> [_ w254]
                tunnel: [w245 w253] -> w237
                frame False {
                }
                frame True {
                  n148 = global read "VAR氨氮全局变量.vi" "状态告警区"() -> (w270:T6)
                  n149 = global read "VAR氨氮全局变量.vi" "状态告警区"() -> (w249:T6)
                  n150 = case shown="\"初始化\"" w251 {
                    selector: w251 -> [w280 _ _]
                    tunnel: [w280 w283 w286] -> w250
                    frame Default {
                    }
                    frame "初始化" {
                      n151 = Concatenate Strings("<<" ("字符串"), "仪器流程开始" ("字符串")) -> (w283:string)
                    }
                    frame "结束" {
                      n152 = Concatenate Strings(">>" ("字符串"), "仪器流程结束" ("字符串")) -> (w286:string)
                    }
                  }
                  n153 = global read "VAR氨氮全局变量.vi" "状态告警区"() -> (w265:T6)
                  n154 = Insert Into Array(array=w255, new element=w254) -> (w253:string[])  [unwired: 1 in]
                  n155 = Unbundle By Name(w270) -> ("id"=w269:u16)
                  n156 = Unbundle By Name(w249) -> ("工作状态"=w248:T8)
                  n157 = Unbundle By Name(w265) -> ("F0"=w262:sgl, "F1"=w261:sgl, "F2"=w260:sgl, "F3"=w259:sgl, "id"=w258:u16, "flowid"=w257:u16, "量程"=w256:u16)
                  n158 = case shown="3, 92" w269 {
                    tunnel: [_ "总磷" ("table输入") "氨氮" ("table输入") "总氮" ("table输入")] -> w267
                    frame Default {
                    }
                    frame 1, 131 {
                    }
                    frame 3, 92 {
                    }
                    frame 2, 76 {
                    }
                  }
                  n159 = case shown="\"水样测试\"" w248 {
                    tunnel: [_ "【水样测试】" ("字符串") "【标样核查】" ("字符串") "【零点核查】" ("字符串") "【跨度核查】" ("字符串") "【空白测试】" ("字符串") "【平行样测试】" ("字符串") "【加标回收】" ("字符串") "【空白校准】" ("字符串") "【标样校准】" ("字符串")] -> w246
                    frame "空闲", Default {
                    }
                    frame "水样测试" {
                    }
                    frame "标样核查" {
                    }
                    frame "零点核查" {
                    }
                    frame "跨度核查" {
                    }
                    frame "空白测试" {
                    }
                    frame "平行样测试" {
                    }
                    frame "加标回收" {
                    }
                    frame "空白校准" {
                    }
                    frame "标样校准" {
                    }
                  }
                  n160 = Format Into String(format string="F0=%#f,F1=%#f,F2=%#f,F3=%#f,Flow=%d-%-d-%-d" ("格式字符串"), w262, w261, w260, w259, w258, w257, w256) -> (resulting string=w263:string)  [unwired: 2 in, 1 out]
                  n161 = Concatenate Strings(w246, w250) -> (w247:string)
                  n162 = Get Date/Time In Seconds() -> (seconds since 1Jan1904=w266:timestamp)
                  n163 = Bundle By Name(cluster=T15 {"时间标识"=timestamp(0 s since 1904-01-01), "设备"="", "日志信息"="", "流程参数"=""} ("data in"), "时间标识"=w266, "设备"=w267, "日志信息"=w247, "流程参数"=w263) -> (w268:T15)
                  n164 = call "氨氮操作日志.vi"("data in"=w268) -> ()  [unwired: 11 in]
                }
              }
            }
            n165 = local write "数组"(w226) -> ()
          }
          frame -1 {
          }
        }
      }
    }
    n166 = call <vilib>:"Boolean Crossing PtByPt.vi"("input"=w166) -> ("crossing"=w130:bool)  [unwired: 2 in]
    n167 = First Call?() -> (First Call?: T/F=w167:bool)
    n168 = case shown="真" w128 {
      tunnel: w124 -> [_ w196]
      tunnel: w123 -> [_ w195]
      frame False {
      }
      frame True {
        n169 = case shown="1, 131" w196 {
          tunnel: [_ "总磷" ("table输入") "氨氮" ("table输入") "总氮" ("table输入")] -> w201
          frame Default {
          }
          frame 1, 131 {
          }
          frame 3, 92 {
          }
          frame 2, 76 {
          }
        }
        n170 = case shown="\"水样测试\"" w195 {
          tunnel: [_ "【水样测试】" ("字符串") "【标样核查】" ("字符串") "【零点核查】" ("字符串") "【跨度核查】" ("字符串") "【空白测试】" ("字符串") "【平行样测试】" ("字符串") "【加标回收】" ("字符串") "【空白校准】" ("字符串") "【标样校准】" ("字符串")] -> w200
          frame "空闲", Default {
          }
          frame "水样测试" {
          }
          frame "标样核查" {
          }
          frame "零点核查" {
          }
          frame "跨度核查" {
          }
          frame "空白测试" {
          }
          frame "平行样测试" {
          }
          frame "加标回收" {
          }
          frame "空白校准" {
          }
          frame "标样校准" {
          }
        }
        n171 = Concatenate Strings("<<" ("字符串"), w200, "启动" ("字符串")) -> (w199:string)
        n172 = Get Date/Time In Seconds() -> (seconds since 1Jan1904=w202:timestamp)
        n173 = Bundle By Name(cluster=T15 {"时间标识"=timestamp(0 s since 1904-01-01), "设备"="", "日志信息"="", "流程参数"=""} ("data in"), "时间标识"=w202, "设备"=w201, "日志信息"=w199) -> (w194:T15)
        n174 = call "氨氮操作日志.vi"("data in"=w194) -> ()  [unwired: 11 in]
      }
    }
    n175 = case shown="真" w125 {
      tunnel: w124 -> [_ w175]
      tunnel: w123 -> [_ w174]
      frame False {
      }
      frame True {
        n176 = case shown="1, 131" w175 {
          tunnel: [_ "总磷" ("table输入") "氨氮" ("table输入") "总氮" ("table输入")] -> w179
          frame Default {
          }
          frame 1, 131 {
          }
          frame 3, 92 {
          }
          frame 2, 76 {
          }
        }
        n177 = case shown="\"水样测试\"" w174 {
          tunnel: [_ "【水样测试】" ("字符串") "【标样核查】" ("字符串") "【零点核查】" ("字符串") "【跨度核查】" ("字符串") "【空白测试】" ("字符串") "【平行样测试】" ("字符串") "【加标回收】" ("字符串") "【空白校准】" ("字符串") "【标样校准】" ("字符串")] -> w178
          frame "空闲", Default {
          }
          frame "水样测试" {
          }
          frame "标样核查" {
          }
          frame "零点核查" {
          }
          frame "跨度核查" {
          }
          frame "空白测试" {
          }
          frame "平行样测试" {
          }
          frame "加标回收" {
          }
          frame "空白校准" {
          }
          frame "标样校准" {
          }
        }
        n178 = Concatenate Strings(w178, "停止" ("字符串"), ">>" ("字符串")) -> (w177:string)
        n179 = Get Date/Time In Seconds() -> (seconds since 1Jan1904=w180:timestamp)
        n180 = Bundle By Name(cluster=T15 {"时间标识"=timestamp(0 s since 1904-01-01), "设备"="", "日志信息"="", "流程参数"=""} ("data in"), "时间标识"=w180, "设备"=w179, "日志信息"=w177) -> (w173:T15)
        n181 = call "氨氮操作日志.vi"("data in"=w173) -> ()  [unwired: 11 in]
      }
    }
    n182 = case shown="真" w168 {
      tunnel: w137 -> [_ w386]
      frame False {
      }
      frame True {
        n183 = Subtract(x=w386, y=1) -> (x-y=w384:i32)
        n184 = Subtract(x=w384, y=5) -> (x-y=w388:i32)
        n185 = Greater Or Equal To 0?(x=w388) -> (x >= 0?=w387:bool)
        n186 = property on="多列列表框" class="MCListbox (严格)"() -> (error out=w392:errorcluster, "TopLeft"=w393:T17)  [unwired: 2 in, 1 out]
        n187 = Select(t=w388, s=w387, f=0) -> (s? t:f=w389:i32)
        n188 = Bundle By Name(cluster=w393, "Row"=w389) -> (w394:T17)
        n189 = property on="多列列表框" class="MCListbox (严格)"(error in=w392, "TopLeft"=w394) -> ()  [unwired: 1 in, 2 out]
      }
    }
    n190 = Or(x=w130, y=w167) -> (x .or. y?=w165:bool)
    n191 = Bundle By Name(cluster=T14 {"启动模式"=enum."跨度核查", "启动参数"=1, "量程"=enum."低量程"} ("参数簇"), "启动参数"=w161, "启动模式"=w163, "量程"=w162) -> (w155:T14)
    n192 = while {
      tunnel: w165 -> [w372]
      tunnel: w155 -> [w371]
      shift-right: [w366] -> _
      shift-left: _ -> [w368]
      shift-right: [w367] -> _
      shift-left: _ -> [w369]
      stop <- TRUE stop-if-true
      n193 = case shown="真" w372 {
        tunnel: [w374 w382] -> w367
        tunnel: [w373 w381] -> w366
        tunnel: w371 -> [_ w376]
        tunnel: w369 -> [w374 _]
        tunnel: w368 -> [w373 _]
        frame False {
        }
        frame True {
          n194 = call "斯坦道XML解析.vi"("添加的路径"="流程路径", "参数簇"=w376) -> ("步骤时间"=w377:string[], "步骤名"=w379:string[])  [unwired: 8 in]
          n195 = Build Array(w379, w377) -> (w378:string[][])
          n196 = for {
            tunnel: w379 -> [_] mode=indexing
            tunnel: [w383] -> w380 mode=indexing
            i -> [w383]
          }
          n197 = Transpose 2D Array(2D array=w378) -> (transposed array=w381:string[][])
          n198 = Number To Decimal String(number=w380) -> (decimal integer string=w382:string[])  [unwired: 1 in]
        }
      }
      n199 = property on="多列列表框" class="MCListbox (严格)"("ItemNames"=w366, "RowHdrs[]"=w367) -> ()  [unwired: 2 in, 2 out]
    }
    n200 = Wait (ms)(milliseconds to wait=u32 1000 ("等待时间（毫秒）")) -> ()  [unwired: 1 out]
  }
  n201 = while {
    tunnel: w22 -> [w400]
    tunnel: w23 -> [_]
    stop <- FALSE stop-if-true
    n202 = Get Queue Status(queue=w400) -> (queue out=w396:refnum<queue>, # elements in queue=w395:i32)  [unwired: 2 in, 6 out]
    n203 = global read "氨氮断电保存全局变量.vi" "MB通信方式选择"() -> (w397:enum16{"串口", "TCP"})
    n204 = global read "氨氮断电保存全局变量.vi" "流程路径"() -> (w399:path)
    n205 = case shown="0" w395 {
      tunnel: w396 -> [_ w406]
      frame Default {
      }
      frame 0 {
        w415 = u16 3 items=["总磷"=1, "氨氮"=3] ("站号")
        # "试剂填充 172 \n管路清洗108\n氨氮92\n总磷131\n总磷海水147\n总氮76\n总氮海水92"
        n206 = global read "VAR氨氮全局变量.vi" "状态告警区"() -> (w407:T6)
        n207 = Unbundle By Name(w407) -> ("系统时间"=w414:timestamp, "工作状态"=w405:T8)
        n208 = Bundle By Name(cluster=cluster{"命令":string, "data":variant} {"命令"="", "data"=variant} ("元素"), "命令"="读状态告警区", "data"=w415) -> (w418:cluster{"命令":string, "data":variant})
        n209 = Get Date/Time In Seconds() -> (seconds since 1Jan1904=w413:timestamp)
        n210 = Enqueue Element(queue=w406, element=w418) -> (queue out=w416:refnum<queue>)  [unwired: 2 in, 2 out]
        n211 = Subtract(x=w413, y=w414) -> (x-y=w412:dbl)
        n212 = Equal?(x=w405, y=T8."空闲") -> (x = y?=w403:bool)
        n213 = Absolute Value(x=w412) -> (abs(x)=w411:dbl)
        n214 = case shown="真" w403 {
          tunnel: w416 -> [w420 w423]
          tunnel: w415 -> [_ w422]
          tunnel: [w420 w421] -> w408
          frame False {
          }
          frame True {
            n215 = Bundle By Name(cluster=cluster{"命令":string, "data":variant} {"命令"="", "data"=variant} ("元素"), "命令"="读测量数据区", "data"=w422) -> (w425:cluster{"命令":string, "data":variant})
            n216 = Enqueue Element(queue=w423, element=w425) -> (queue out=w421:refnum<queue>)  [unwired: 2 in, 2 out]
          }
        }
        n217 = Greater Or Equal?(x=w411, y=120.0) -> (x >= y?=w409:bool)
        n218 = case shown="真" w409 {
          tunnel: w408 -> [_ w428]
          frame False {
          }
          frame True {
            n219 = call "氨氮启动命令.vi"("参数"=T18 {"站号"=3, "量程切换"=enum."AUTO", "控制命令"=enum."校时", "模式设置"=enum."待机", "测量间隔"=0}) -> ("启动命令"=w427:cluster{"命令":string, "data":variant})  [unwired: 10 in]
            n220 = Enqueue Element(queue=w428, element=w427) -> ()  [unwired: 2 in, 3 out]
          }
        }
      }
    }
    n221 = case shown="\"TCP\"" w397 {
      tunnel: [w430 w431] -> w398
      frame "串口", Default {
        n222 = global read "氨氮断电保存全局变量.vi" "VISA Resource"() -> (w430:refnum<visa-resource-name>)
      }
      frame "TCP" {
        n223 = global read "氨氮断电保存全局变量.vi" "IP"() -> (w431:string)
      }
    }
    "字符串" <- w398
    n224 = local write "流程路径"(w399) -> ()
    n225 = Wait (ms)(milliseconds to wait=u32 1000 ("等待时间（毫秒）")) -> ()  [unwired: 1 out]
  }
  n226 = while {
    tunnel: w22 -> [w439]
    tunnel: w21 -> [w438]
    tunnel: w20 -> [w437]
    tunnel: w19 -> [w436]
    tunnel: w18 -> [w435]
    tunnel: w17 -> [w434]
    tunnel: w16 -> [w433]
    tunnel: w11 -> [_]
    tunnel: w7 -> [w432]
    stop <- FALSE stop-if-true
    n227 = event shown="[9] \"仪器参数设置\": 值改变" {
      selector: _ -> [_ _ _ _ _ _ _ _ _ _ _ _ _ _ _ _ _ _ _ _ _ _ _]
      dyn-events: _ -> [_ _ _ _ _ _ _ _ _ _ _ _ _ _ _ _ _ _ _ _ _ _ _]
      timeout: _ -> [_ _ _ _ _ _ _ _ _ _ _ _ _ _ _ _ _ _ _ _ _ _ _]
      tunnel: w439 -> [_ _ w455 w483 _ _ _ _ _ _ _ w591 w600 w607 _ _ _ _ _ _ _ _ _]
      tunnel: w438 -> [_ _ _ _ _ _ _ _ _ _ _ _ _ _ _ _ _ w623 _ w657 w666 w672 w684]
      tunnel: w437 -> [_ _ _ _ _ _ _ _ _ _ _ _ _ _ _ _ _ w621 _ w655 w668 w680 w691]
      tunnel: w436 -> [_ _ _ _ _ _ _ _ _ _ _ _ _ _ _ _ _ w622 _ w656 w667 w674 w686]
      tunnel: w435 -> [_ _ _ _ _ _ _ _ _ _ _ _ _ _ _ _ _ w617 _ _ _ _ _]
      tunnel: w434 -> [_ _ _ _ _ _ _ _ _ _ _ _ _ _ _ _ _ _ _ w651 _ _ _]
      tunnel: w433 -> [_ _ _ _ _ _ _ _ _ _ _ _ _ _ _ _ _ _ _ _ _ w678 _]
      tunnel: w432 -> [_ _ _ _ _ _ _ _ _ _ _ _ _ w603 _ _ _ _ _ _ _ _ _]
      tunnel: [_ w441 _ _ _ _ _ _ _ _ _ _ _ _ _ _ _ _ _ _ _ _ _] -> _
      event Timeout {
        n228 = event-data() -> ()  [unwired: 1 in, 3 out]
      }
      event "测量模式下拉列表", "量程下拉列表", "参数下拉列表": Value Change {
        n229 = event-data() -> ()  [unwired: 1 in, 6 out]
        n230 = local read "参数下拉列表"() -> (w442:enum16{"总磷", "总氮", "氨氮"})
        n231 = local read "测量模式下拉列表"() -> (w443:enum16{"水样测量", "零点核查", "跨度核查", "标样核查", "加标回收"})
        n232 = local read "量程下拉列表"() -> (w444:enum16{"低量程", "高量程"})
        n233 = Bundle("参数下拉列表"=w442, "测量模式下拉列表"=w443, "量程下拉列表"=w444) -> (w445:T13)  [unwired: 1 in]
        n234 = property on="曲线模型" class="曲线模型 (严格)"("属性"=w445) -> (error out=w441:errorcluster)  [unwired: 2 in, 1 out]
      }
      event "串口设置": Value Change {
        n235 = event-data() -> ()  [unwired: 1 in, 6 out]
        n236 = global read "氨氮断电保存全局变量.vi" "VISA Resource"() -> (w452:refnum<visa-resource-name>)
        n237 = global read "氨氮断电保存全局变量.vi" "MB通信方式选择"() -> (w446:enum16{"串口", "TCP"})
        n238 = global read "氨氮断电保存全局变量.vi" "IP"() -> (w451:string)
        n239 = global read "氨氮断电保存全局变量.vi" "PORT"() -> (w450:string)
        n240 = call "串口配置.vi"("PORT"=w450, "IP"=w451, "MB通信方式选择"=w446, "请选择串口:"=w452) -> ("PORT 2"=w448:string, "IP 2"=w449:string, "确认 2"=w453:bool, "VISA资源名称 2"=w454:refnum<visa-resource-name>, "MB通信方式选择 2"=w447:enum16{"串口", "TCP"})  [unwired: 3 in]
        n241 = case shown="真" w453 {
          tunnel: w454 -> [_ w460]
          tunnel: w455 -> [_ w459]
          tunnel: w449 -> [_ w458]
          tunnel: w448 -> [_ w457]
          tunnel: w447 -> [_ w456]
          frame False {
          }
          frame True {
            n242 = flat-sequence {
              tunnel: w460 -> [w465]
              tunnel: w459 -> [w466]
              tunnel: w458 -> [w464]
              tunnel: w457 -> [w463]
              tunnel: w456 -> [w462]
              frame #0 {
                n243 = global write "氨氮断电保存全局变量.vi" "VISA Resource"(w465) -> ()
                n244 = global write "氨氮断电保存全局变量.vi" "IP"(w464) -> ()
                n245 = global write "氨氮断电保存全局变量.vi" "PORT"(w463) -> ()
                n246 = global write "氨氮断电保存全局变量.vi" "MB通信方式选择"(w462) -> ()
                n247 = Flush Queue(queue=w466) -> (queue out=w461:refnum<queue>)  [unwired: 1 in, 2 out]
                n248 = Enqueue Element(queue=w461, element=cluster{"命令":string, "data":variant} {"命令"="启用模块", "data"=variant} ("元素")) -> ()  [unwired: 2 in, 3 out]
              }
              frame #1 {
                n249 = call <vilib>:"Application Directory.vi"() -> ("Application Directory"=w481:path)
                n250 = Build Path(base path=w481, name or relative path="data\\sys.ini" ("名称或相对路径")) -> (appended path=w479:path)
                n251 = call <vilib>:"Open Config Data.vi"("configuration file path"=w479) -> ("error out"=w475:errorcluster, "refnum"=w478:T12)  [unwired: 8 in, 1 out]
                n252 = vi-ref "氨氮断电保存全局变量.vi"() -> (w477:refnum<vi>)
                n253 = call <userlib>:"Write Panel to INI__ogtk.vi"("error in (no error)"=w475, "VI ref"=w477, "refnum"=w478) -> ("error out"=w474:errorcluster, "refnum out"=w476:T12)  [unwired: 7 in]
                n254 = call <vilib>:"Close Config Data.vi"("error in (no error)"=w474, "refnum"=w476) -> ("error out"=w469:errorcluster, "file path"=w468:path)  [unwired: 8 in]
                n255 = Open/Create/Replace File(file path (use dialog)=w468, error in=w469) -> (refnum out=w472:refnum<file>, error out=w473:errorcluster)  [unwired: 4 in, 1 out]
                n256 = Flush File(refnum=w472, error in=w473) -> (refnum out=w471:refnum<file>, error out=w470:errorcluster)
                n257 = Close File(refnum=w471, error in=w470) -> ()  [unwired: 2 out]
              }
            }
          }
        }
      }
      event "模块启用": Value Change {
        n258 = event-data() -> ("OldVal"=w484:bool)  [unwired: 1 in, 5 out]
        n259 = Flush Queue(queue=w483) -> (queue out=w482:refnum<queue>)  [unwired: 1 in, 2 out]
        n260 = case shown="假" w484 {
          tunnel: w482 -> [w485 w487]
          frame False {
            n261 = Enqueue Element(queue=w485, element=cluster{"命令":string, "data":variant} {"命令"="停用模块", "data"=variant} ("元素")) -> ()  [unwired: 2 in, 3 out]
          }
          frame True {
            n262 = Enqueue Element(queue=w487, element=cluster{"命令":string, "data":variant} {"命令"="启用模块", "data"=variant} ("元素")) -> ()  [unwired: 2 in, 3 out]
          }
        }
      }
      event "流程路径": Value Change {
        n263 = event-data() -> ()  [unwired: 1 in, 6 out]
        n264 = flat-sequence {
          frame #0 {
            n265 = local read "流程路径"() -> (w489:path)
            n266 = global write "氨氮断电保存全局变量.vi" "流程路径"(w489) -> ()
          }
          frame #1 {
            n267 = call <vilib>:"Application Directory.vi"() -> ("Application Directory"=w503:path)
            n268 = Build Path(base path=w503, name or relative path="data\\sys.ini" ("名称或相对路径")) -> (appended path=w501:path)
            n269 = call <vilib>:"Open Config Data.vi"("configuration file path"=w501) -> ("error out"=w497:errorcluster, "refnum"=w500:T12)  [unwired: 8 in, 1 out]
            n270 = vi-ref "氨氮断电保存全局变量.vi"() -> (w499:refnum<vi>)
            n271 = call <userlib>:"Write Panel to INI__ogtk.vi"("error in (no error)"=w497, "VI ref"=w499, "refnum"=w500) -> ("error out"=w496:errorcluster, "refnum out"=w498:T12)  [unwired: 7 in]
            n272 = call <vilib>:"Close Config Data.vi"("error in (no error)"=w496, "refnum"=w498) -> ("error out"=w491:errorcluster, "file path"=w490:path)  [unwired: 8 in]
            n273 = Open/Create/Replace File(file path (use dialog)=w490, error in=w491) -> (refnum out=w494:refnum<file>, error out=w495:errorcluster)  [unwired: 4 in, 1 out]
            n274 = Flush File(refnum=w494, error in=w495) -> (refnum out=w493:refnum<file>, error out=w492:errorcluster)
            n275 = Close File(refnum=w493, error in=w492) -> ()  [unwired: 2 out]
          }
        }
      }
      event "公式一键写入": Value Change {
        n276 = event-data() -> ()  [unwired: 1 in, 6 out]
        n277 = local read "公式"() -> (w504:cluster{"X^2":dbl, "X":dbl, "b":dbl})
        n278 = call "公式复合写入.vi"("公式"=w504) -> ()  [unwired: 11 in]
      }
      event "备用系数一键写入": Value Change {
        n279 = event-data() -> ()  [unwired: 1 in, 6 out]
        n280 = local read "备用系数"() -> (w505:T4)
        n281 = call "量程参数复合参数写入.vi"("备用系数"=w505) -> ()  [unwired: 11 in]
      }
      event "曲线模型": Value Change {
        n282 = event-data() -> ()  [unwired: 1 in, 6 out]
        n283 = Unbundle By Name("曲线模型") -> ("X^2"=w508:dbl, "X"=w507:dbl, "B"=w506:dbl)
        n284 = local read "公式"() -> (w511:cluster{"X^2":dbl, "X":dbl, "b":dbl})
        n285 = Bundle By Name(cluster=w511, "X^2"=w508, "X"=w507, "b"=w506) -> (w510:cluster{"X^2":dbl, "X":dbl, "b":dbl})
        n286 = local write "公式"(w510) -> ()
      }
      event "质控参数设置": Value Change {
        n287 = event-data() -> ()  [unwired: 1 in, 6 out]
        n288 = global read "氨氮断电保存全局变量.vi" "质控参数设置"() -> (w512:T19)
        n289 = call "氨氮质控参数设置.vi"("质控参数设置"=w512) -> ("输出簇"=w513:T20)  [unwired: 10 in]
        n290 = Unbundle By Name(w513) -> ("确定"=w514:bool)
        n291 = case shown="真" w514 {
          tunnel: w513 -> [_ w516]
          tunnel: w512 -> [_ w515]
          frame False {
          }
          frame True {
            n292 = flat-sequence {
              tunnel: w516 -> [w523]
              tunnel: w515 -> [w522]
              frame #0 {
                n293 = Unbundle By Name(w523) -> ("跨度值"=w521:dbl, "零点标准液浓度"=w520:dbl, "跨度标准液浓度"=w519:dbl, "标准液标准浓度"=w518:dbl)
                n294 = Bundle By Name(cluster=w522, "氨氮跨度值"=w521, "氨氮零点标准液浓度"=w520, "氨氮跨度标准液浓度"=w519, "氨氮标准液标准浓度"=w518) -> (w517:T19)
                n295 = global write "氨氮断电保存全局变量.vi" "质控参数设置"(w517) -> ()
              }
              frame #1 {
                n296 = call <vilib>:"Application Directory.vi"() -> ("Application Directory"=w537:path)
                n297 = Build Path(base path=w537, name or relative path="data\\sys.ini" ("名称或相对路径")) -> (appended path=w535:path)
                n298 = call <vilib>:"Open Config Data.vi"("configuration file path"=w535) -> ("error out"=w531:errorcluster, "refnum"=w534:T12)  [unwired: 8 in, 1 out]
                n299 = vi-ref "氨氮断电保存全局变量.vi"() -> (w533:refnum<vi>)
                n300 = call <userlib>:"Write Panel to INI__ogtk.vi"("error in (no error)"=w531, "VI ref"=w533, "refnum"=w534) -> ("error out"=w530:errorcluster, "refnum out"=w532:T12)  [unwired: 7 in]
                n301 = call <vilib>:"Close Config Data.vi"("error in (no error)"=w530, "refnum"=w532) -> ("error out"=w525:errorcluster, "file path"=w524:path)  [unwired: 8 in]
                n302 = Open/Create/Replace File(file path (use dialog)=w524, error in=w525) -> (refnum out=w528:refnum<file>, error out=w529:errorcluster)  [unwired: 4 in, 1 out]
                n303 = Flush File(refnum=w528, error in=w529) -> (refnum out=w527:refnum<file>, error out=w526:errorcluster)
                n304 = Close File(refnum=w527, error in=w526) -> ()  [unwired: 2 out]
              }
            }
          }
        }
      }
      event "仪器参数设置": Value Change {
        n305 = event-data() -> ()  [unwired: 1 in, 6 out]
        n306 = global read "氨氮断电保存全局变量.vi" "氨氮仪器参数"() -> (w539:T21)
        n307 = call "仪器参数设置.vi"("氨氮仪器参数"=w539) -> ("仪器参数设置输出"=w538:T22)  [unwired: 10 in]
        n308 = Unbundle By Name(w538) -> ("确定"=w540:bool)
        n309 = case shown="真" w540 {
          tunnel: w538 -> [_ w542]
          tunnel: w539 -> [_ w541]
          frame False {
          }
          frame True {
            n310 = flat-sequence {
              tunnel: w542 -> [w559]
              tunnel: w541 -> [w558]
              frame #0 {
                n311 = Unbundle By Name(w559) -> ("测量量程"=w557:dbl, "测量精度"=w556:dbl, "测量间隔"=w555:dbl, "消解温度"=w554:dbl, "消解时长"=w552:dbl, "空白校准时间"=w551:timestamp, "曲线截距"=w550:dbl, "曲线斜率"=w549:dbl, "测量检出限"=w548:dbl, "测量信号值"=w547:dbl, "线性相关系数"=w546:dbl, "二次多项式系数"=w545:dbl, "标样校准时间"=w544:timestamp, "稀释倍数"=w543:dbl)
                n312 = Bundle By Name(cluster=w558, "测量量程"=w557, "测量精度"=w556, "测量间隔"=w555, "消解温度"=w554, "消解时长"=w552, "空白校准时间"=w551, "曲线截距"=w550, "曲线斜率"=w549, "测量检出限"=w548, "测量信号值"=w547, "线性相关系数"=w546, "二次多项式系数"=w545, "标样校准时间"=w544, "稀释倍数"=w543) -> (w553:T21)
                n313 = global write "氨氮断电保存全局变量.vi" "氨氮仪器参数"(w553) -> ()
              }
              frame #1 {
                n314 = call <vilib>:"Application Directory.vi"() -> ("Application Directory"=w573:path)
                n315 = Build Path(base path=w573, name or relative path="data\\sys.ini" ("名称或相对路径")) -> (appended path=w571:path)
                n316 = call <vilib>:"Open Config Data.vi"("configuration file path"=w571) -> ("error out"=w567:errorcluster, "refnum"=w570:T12)  [unwired: 8 in, 1 out]
                n317 = vi-ref "氨氮断电保存全局变量.vi"() -> (w569:refnum<vi>)
                n318 = call <userlib>:"Write Panel to INI__ogtk.vi"("error in (no error)"=w567, "VI ref"=w569, "refnum"=w570) -> ("error out"=w566:errorcluster, "refnum out"=w568:T12)  [unwired: 7 in]
                n319 = call <vilib>:"Close Config Data.vi"("error in (no error)"=w566, "refnum"=w568) -> ("error out"=w561:errorcluster, "file path"=w560:path)  [unwired: 8 in]
                n320 = Open/Create/Replace File(file path (use dialog)=w560, error in=w561) -> (refnum out=w564:refnum<file>, error out=w565:errorcluster)  [unwired: 4 in, 1 out]
                n321 = Flush File(refnum=w564, error in=w565) -> (refnum out=w563:refnum<file>, error out=w562:errorcluster)
                n322 = Close File(refnum=w563, error in=w562) -> ()  [unwired: 2 out]
              }
            }
          }
        }
      }
      event "自动测试量程配置": Value Change {
        n323 = event-data() -> ()  [unwired: 1 in, 6 out]
        n324 = flat-sequence {
          frame #0 {
            n325 = global write "氨氮断电保存全局变量.vi" "氨氮自动测试量程配置"("自动测试量程配置") -> ()
          }
          frame #1 {
            n326 = call <vilib>:"Application Directory.vi"() -> ("Application Directory"=w588:path)
            n327 = Build Path(base path=w588, name or relative path="data\\sys.ini" ("名称或相对路径")) -> (appended path=w586:path)
            n328 = call <vilib>:"Open Config Data.vi"("configuration file path"=w586) -> ("error out"=w582:errorcluster, "refnum"=w585:T12)  [unwired: 8 in, 1 out]
            n329 = vi-ref "氨氮断电保存全局变量.vi"() -> (w584:refnum<vi>)
            n330 = call <userlib>:"Write Panel to INI__ogtk.vi"("error in (no error)"=w582, "VI ref"=w584, "refnum"=w585) -> ("error out"=w581:errorcluster, "refnum out"=w583:T12)  [unwired: 7 in]
            n331 = call <vilib>:"Close Config Data.vi"("error in (no error)"=w581, "refnum"=w583) -> ("error out"=w576:errorcluster, "file path"=w575:path)  [unwired: 8 in]
            n332 = Open/Create/Replace File(file path (use dialog)=w575, error in=w576) -> (refnum out=w579:refnum<file>, error out=w580:errorcluster)  [unwired: 4 in, 1 out]
            n333 = Flush File(refnum=w579, error in=w580) -> (refnum out=w578:refnum<file>, error out=w577:errorcluster)
            n334 = Close File(refnum=w578, error in=w577) -> ()  [unwired: 2 out]
          }
        }
      }
      event "手动启动": Value Change {
        n335 = event-data() -> ()  [unwired: 1 in, 6 out]
        n336 = call "氨氮启动参数对话框.vi"() -> ("确认"=w589:bool, "元素"=w590:cluster{"命令":string, "data":variant})  [unwired: 10 in]
        n337 = case shown="真" w589 {
          tunnel: w591 -> [_ w593]
          tunnel: w590 -> [_ w592]
          frame False {
          }
          frame True {
            n338 = Enqueue Element(queue=w593, element=w592) -> ()  [unwired: 2 in, 3 out]
          }
        }
      }
      event "单步测试": Value Change {
        w595 = u16 1 items=["总磷"=1, "氨氮"=3] ("站号")
        n339 = event-data() -> ()  [unwired: 1 in, 6 out]
        n340 = Bundle("站号"=w595, "总磷氨氮调试"="总磷氨氮调试") -> (w594:cluster{"站号":u16, "总磷氨氮调试":u16[]})  [unwired: 1 in]
        n341 = Bundle By Name(cluster=cluster{"命令":string, "data":variant} {"命令"="", "data"=variant} ("元素"), "命令"="debug", "data"=w594) -> (w597:cluster{"命令":string, "data":variant})
        n342 = Enqueue Element(queue=w600, element=w597) -> ()  [unwired: 2 in, 3 out]
      }
      event "停止": Value Change {
        n343 = event-data() -> ()  [unwired: 1 in, 6 out]
        n344 = Cancel Notification(0:w603) -> (8:w604:refnum<notifier>)  [unwired: 1 in, 2 out]
        n345 = Enqueue Element(queue=w607, element=cluster{"命令":string, "data":variant} {"命令"="启动", "data"=variant(cluster{"站号":u16, "控制命令输出":u16[]} {"站号"=1, "控制命令输出"=[2816]})} ("元素")) -> (queue out=w605:refnum<queue>)  [unwired: 2 in, 2 out]
        n346 = Send Notification(notification=TRUE ("通知"), notifier=w604) -> ()  [unwired: 1 in, 2 out]
        n347 = Enqueue Element(queue=w605, element=cluster{"命令":string, "data":variant} {"命令"="启动", "data"=variant(cluster{"站号":u16, "控制命令":u16[]} {"站号"=3, "控制命令"=[2816]})} ("启动命令")) -> ()  [unwired: 2 in, 3 out]
      }
      event "设置": Value Change {
        n348 = event-data() -> ()  [unwired: 1 in, 6 out]
        n349 = property on="窗格" class="Pane"("Origin"=T10 {"Horizontal"=0, "Vertical"=628} ("原点")) -> ()  [unwired: 2 in, 2 out]
      }
      event "返回": Value Change {
        n350 = event-data() -> ()  [unwired: 1 in, 6 out]
        n351 = property on="窗格" class="Pane"("Origin"=T10 {"Horizontal"=0, "Vertical"=0} ("原点")) -> ()  [unwired: 2 in, 2 out]
      }
      event "公式.X^2", "公式.X", "公式.b", "量程切换阈值.阈值", "量程切换阈值.标液浓度", "备用系数.量程上限", "备用系数.量程下限", "备用系数.检出限", "备用系数.精度": Mouse Down {
        n352 = event-data() -> ("CtlRef"=w613:refnum<vi>)  [unwired: 1 in, 5 out]
        n353 = property class="DigNum (严格)"(reference=w613) -> (reference out=w611:refnum<vi>, "Value"=w612:dbl)  [unwired: 1 in, 1 out]
        n354 = call "数字键盘.vi"("OldNumber"=w612) -> ("NewNumber"=w610:dbl)
        n355 = property class="DigNum (严格)"(reference=w611, "Val(Sgnl)"=w610) -> ()  [unwired: 1 in, 2 out]
      }
      event "读公式": Value Change {
        n356 = event-data() -> ()  [unwired: 1 in, 6 out]
        n357 = property class="Enum (严格)"(reference=w621) -> ("Value"=w620:enum16{"总磷", "总氮", "氨氮"})  [unwired: 1 in, 2 out]
        n358 = property class="Enum (严格)"(reference=w622) -> ("Value"=w619:enum16{"水样测量", "零点核查", "跨度核查", "标样核查", "加标回收"})  [unwired: 1 in, 2 out]
        n359 = property class="Enum (严格)"(reference=w623) -> ("Value"=w618:enum16{"低量程", "高量程"})  [unwired: 1 in, 2 out]
        n360 = call "公式读取.vi"("量程"=w618, "测量模式"=w619, "测量参数"=w620) -> ("error out"=w615:errorcluster, "公式"=w616:cluster{"X^2":dbl, "X":dbl, "b":dbl})  [unwired: 7 in]
        n361 = property class="Clust (严格)"(reference=w617, "Value"=w616) -> ()  [unwired: 1 in, 2 out]
        n362 = case shown="错误" w615 {
          tunnel: ["读取成功" ("消息") "读取失败" ("消息")] -> w614
          frame No Error {
          }
          frame Error {
          }
        }
        n363 = One Button Dialog(message=w614) -> ()  [unwired: 1 in, 1 out]
      }
      event "写公式": Value Change {
        n364 = event-data() -> ()  [unwired: 1 in, 6 out]
        n365 = call "公式写入.vi"("公式"="公式", "量程"="量程下拉列表", "测量模式"="测量模式下拉列表", "测量参数"="参数下拉列表") -> ("error out"=w630:errorcluster)  [unwired: 7 in]
        n366 = case shown="无错误" w630 {
          tunnel: ["写入成功" ("消息") "写入失败" ("消息")] -> w631
          tunnel: "测量模式下拉列表" -> [w637 _]
          tunnel: "量程下拉列表" -> [w636 _]
          tunnel: "公式" -> [w632 _]
          frame No Error {
            n367 = Equal?(x=w637, y=enum16{"水样测量", "零点核查", "跨度核查", "标样核查", "加标回收"}."水样测量") -> (x = y?=w635:bool)
            n368 = Equal?(x=w636, y=enum16{"低量程", "高量程"}."低量程") -> (x = y?=w634:bool)
            n369 = And(x=w635, y=w634) -> (x .and. y?=w633:bool)
            n370 = case shown="真" w633 {
              tunnel: w632 -> [_ w641]
              frame False {
              }
              frame True {
                n371 = Unbundle By Name(w641) -> ("X^2"=w644:dbl, "X"=w643:dbl, "b"=w642:dbl)
                n372 = global read "氨氮断电保存全局变量.vi" "氨氮仪器参数"() -> (w645:T21)
                n373 = Bundle By Name(cluster=w645, "曲线截距"=w642, "曲线斜率"=w643, "二次多项式系数"=w644) -> (w646:T21)
                n374 = global write "氨氮断电保存全局变量.vi" "氨氮仪器参数"(w646) -> ()
              }
            }
          }
          frame Error {
          }
        }
        n375 = One Button Dialog(message=w631) -> ()  [unwired: 1 in, 1 out]
      }
      event "量程切换阈值读取": Value Change {
        n376 = event-data() -> ()  [unwired: 1 in, 6 out]
        n377 = property class="Enum (严格)"(reference=w655) -> ("Value"=w654:enum16{"总磷", "总氮", "氨氮"})  [unwired: 1 in, 2 out]
        n378 = property class="Enum (严格)"(reference=w656) -> ("Value"=w653:enum16{"水样测量", "零点核查", "跨度核查", "标样核查", "加标回收"})  [unwired: 1 in, 2 out]
        n379 = property class="Enum (严格)"(reference=w657) -> ("Value"=w652:enum16{"低量程", "高量程"})  [unwired: 1 in, 2 out]
        n380 = call "量程读取.vi"("量程"=w652, "测量模式"=w653, "测量参数"=w654) -> ("error out"=w648:errorcluster, "量程切换阈值"=w650:cluster{"阈值":dbl, "标液浓度":dbl})  [unwired: 7 in]
        n381 = property class="Clust (严格)"(reference=w651, "Value"=w650) -> ()  [unwired: 1 in, 2 out]
        n382 = case shown="错误" w648 {
          tunnel: ["读取成功" ("消息") "读取失败" ("消息")] -> w649
          frame No Error {
          }
          frame Error {
          }
        }
        n383 = One Button Dialog(message=w649) -> ()  [unwired: 1 in, 1 out]
      }
      event "量程切换阈值写入": Value Change {
        n384 = event-data() -> ()  [unwired: 1 in, 6 out]
        n385 = property class="Enum (严格)"(reference=w668) -> ("Value"=w665:enum16{"总磷", "总氮", "氨氮"})  [unwired: 1 in, 2 out]
        n386 = property class="Enum (严格)"(reference=w667) -> ("Value"=w664:enum16{"水样测量", "零点核查", "跨度核查", "标样核查", "加标回收"})  [unwired: 1 in, 2 out]
        n387 = property class="Enum (严格)"(reference=w666) -> ("Value"=w663:enum16{"低量程", "高量程"})  [unwired: 1 in, 2 out]
        n388 = call "量程写入.vi"("量程切换阈值"="量程切换阈值", "量程"=w663, "测量模式"=w664, "测量参数"=w665) -> ("error out"=w660:errorcluster)  [unwired: 7 in]
        n389 = case shown="无错误" w660 {
          tunnel: ["写入成功" ("消息") "写入失败" ("消息")] -> w661
          frame No Error {
          }
          frame Error {
          }
        }
        n390 = One Button Dialog(message=w661) -> ()  [unwired: 1 in, 1 out]
      }
      event "备用系数读取": Value Change {
        n391 = event-data() -> ()  [unwired: 1 in, 6 out]
        n392 = property class="Enum (严格)"(reference=w680) -> ("Value"=w679:enum16{"总磷", "总氮", "氨氮"})  [unwired: 1 in, 2 out]
        n393 = property class="Enum (严格)"(reference=w674) -> ("Value"=w673:enum16{"水样测量", "零点核查", "跨度核查", "标样核查", "加标回收"})  [unwired: 1 in, 2 out]
        n394 = property class="Enum (严格)"(reference=w672) -> ("Value"=w671:enum16{"低量程", "高量程"})  [unwired: 1 in, 2 out]
        n395 = call "备用系数读取.vi"("量程"=w671, "测量模式"=w673, "测量参数"=w679) -> ("error out"=w675:errorcluster, "备用系数"=w677:T4)  [unwired: 7 in]
        n396 = property class="Clust (严格)"(reference=w678, "Value"=w677) -> ()  [unwired: 1 in, 2 out]
        n397 = case shown="错误" w675 {
          tunnel: ["读取成功" ("消息") "读取失败" ("消息")] -> w676
          frame No Error {
          }
          frame Error {
          }
        }
        n398 = One Button Dialog(message=w676) -> ()  [unwired: 1 in, 1 out]
      }
      event "备用系数写入": Value Change {
        n399 = event-data() -> ()  [unwired: 1 in, 6 out]
        n400 = property class="Enum (严格)"(reference=w691) -> ("Value"=w690:enum16{"总磷", "总氮", "氨氮"})  [unwired: 1 in, 2 out]
        n401 = property class="Enum (严格)"(reference=w686) -> ("Value"=w685:enum16{"水样测量", "零点核查", "跨度核查", "标样核查", "加标回收"})  [unwired: 1 in, 2 out]
        n402 = property class="Enum (严格)"(reference=w684) -> ("Value"=w683:enum16{"低量程", "高量程"})  [unwired: 1 in, 2 out]
        n403 = call "备用系数写入.vi"("备用系数"="备用系数", "量程"=w683, "测量模式"=w685, "测量参数"=w690) -> ("error out"=w687:errorcluster)  [unwired: 7 in]
        n404 = case shown="无错误" w687 {
          tunnel: ["写入成功" ("消息") "写入失败" ("消息")] -> w688
          frame No Error {
          }
          frame Error {
          }
        }
        n405 = One Button Dialog(message=w688) -> ()  [unwired: 1 in, 1 out]
      }
    }
  }
  n406 = while {
    stop <- FALSE stop-if-true
    n407 = Wait (ms)(milliseconds to wait=u32 1000 ("等待时间（毫秒）")) -> ()  [unwired: 1 out]
    n408 = global read "系统设置全局变量.vi" "三级权限"() -> (w697:bool)
    n409 = Select(t=T23."Enabled" ("禁用"), s=w697, f=T23."Disabled and Grayed Out" ("禁用")) -> (s? t:f=w694:T23)
    n410 = property on="设置" class="Bool"("DisabledEnum"=w694) -> ()  [unwired: 2 in, 2 out]
  }
